vi "LogLoop_HDF5_20190307.vi"(8 "error in":errorcluster, 11 "Queue in":refnum<queue>) -> (0 "error out":errorcluster)   [LabVIEW 2018]
uses:
  Controls/Enums/LogLoopEnum.ctl
  Controls/Clusts/LogLoopClust.ctl
  Controls/Clusts/Config_Clust.ctl
  Controls/Clusts/UserConfig.ctl
  Controls/PathsCluster.ctl
  Controls/Clusts/FrontPanel_UserConfig.ctl
  Controls/Clusts/Inclinometer_User_Cfg.ctl
  Controls/Clusts/FP_UserTargetConfig.ctl
  Controls/Clusts/FreqShift.ctl
  Controls/Clusts/FPGA_Scale.ctl
  Controls/Enums/ScaleMeasure.ctl
  Controls/RadioButtons/FilterEnableRadio.ctl
  Controls/Enums/TargetNumber.ctl
  Controls/Clusts/HDF5_File_Refs.ctl
  <vilib>/addons/h5labview2/base/hid_t.ctl
  Controls/Clusts/ToneGroupRefsClust.ctl
  HDF5/HDF5_Tone_refs.ctl
  HDF5/HDF5_Noise_refs.ctl
  HDF5/TC_Tone_refs.ctl
  HDF5/HDF5_Validty_refs.ctl
  HDF5/HDF5_Disdrometer_Refs.ctl
  HDF5/HDF5_Health_Refs.ctl
  HDF5/UPS_refs.ctl
  Controls/Clusts/WeatherRefs.ctl
  HDF5/HDF5_AI_refs.ctl
  HDF5/HDF5_Filter_refs.ctl
  HDF5/HDF5_ADAM_Refs.ctl
  HDF5/HDF5_Complex_Refs.ctl
  Controls/Clusts/LogDataClust.ctl
  Controls/Clusts/ToneLogBuffered.ctl
  Controls/Clusts/SaturationMonitorBuffer.ctl
  HDF5/TC_Data_Structure.ctl
  Controls/Clusts/AI_Clust.ctl
  HDF5/HDF5_NoiseInfoClust.ctl
  HDF5/DisdrometerData.ctl
  HDF5/DisdromterSummaryData.ctl
  Disdrometer/Disdrometer_Status_Cluster.ctl
  Controls/Clusts/WeatherDataClust.ctl
  Controls/Clusts/ValidityWeatherClust.ctl
  Controls/Clusts/TE_Data_Clust.ctl
  HDF5/HDF5_ADAM_Data.ctl
  Controls/Clusts/TimeDomainData.ctl
  Controls/Clusts/AlarmSettingsClust.ctl
  Controls/Clusts/AlarmThresh_OneChan.ctl
  Controls/Clusts/ErrorStatus.ctl
  Controls/Clusts/DigOutClust.ctl
  Controls/Clusts/Saturation_Status_Clust.ctl
  Controls/Clusts/HDF5_10HzRefs.ctl
  Controls/Clusts/TargetToneData.ctl
  Controls/Clusts/ChannelToneData.ctl
  Controls/ToneInfoClust.ctl
  Controls/Clusts/SaturationMonitor.ctl
  Controls/Clusts/All_TC_Error_and_Data.ctl
  Controls/Clusts/All_TC_Error_Status.ctl
  Controls/Clusts/All_AI_Error_and_Data.ctl
  Controls/Clusts/All_AI_Error_Status.ctl
  Controls/Clusts/UPS_Status_Clust.ctl
  Controls/Enums/FP_Loop_Enum.ctl
  Controls/Enums/DigiLoopEnum.ctl
  Controls/Enums/WatchdogTimer_Enum.ctl
  <vilib>/addons/h5labview2/file/H5F.lvlib
panel:
  out "base path 2":path
  out "WatchDogElapsed":i32[](array[numeric])
  out "Elapsed":u32
  out "#LogElements":i32
  out "LogCount":i32
  out "LogState":T1
  out "date/time string":string
  out "Enum":T1
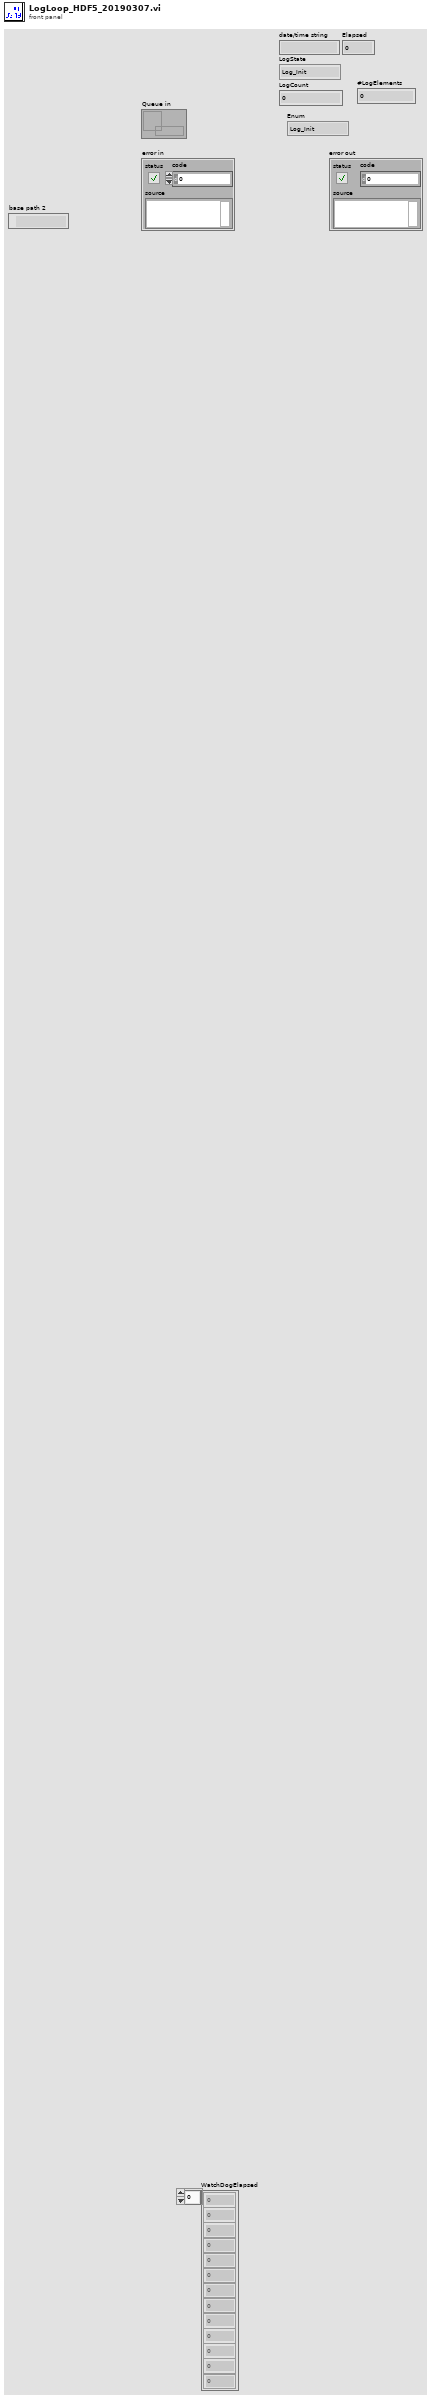
[diagram p1: front panel]
types:
  T1 = typedef "LogLoopEnum.ctl" = enum16{"Log_Init", "Log_Config", "Log_CfgAlarm", "Log_TimeDomain", "Log_Tone", "Log_NoiseTrace", "Log_NoiseSum", "Log_DO", "Log_AI", "Log_TC", "Log_Disdrom", "Log_Weather", "Log_TE", "Log_ADAM", "Log_UPS", "Log_ChkTime", "Log_Alarm", "Log_SSH", "Log_Write", "Log_Exit"}
  T2 = typedef "LogLoopClust.ctl" = cluster{"base path":path, "PathNow1":path, "PathNow2":path, "DateNow":string, "NAS path":path, "LogFiltStage":bool, "LogNoise_df_1":bool, "LogNoise_df_2":bool, "LogNoise_df_3":bool, "LogNoise_df_4":bool, "Config":T3, "HDFRefs1":T14, "HDFRefs2":T14, "LogData":T29, "AlarmCfg":T43, "DO":bool[], "AllAlarms":T45[], "Alarm Status":T46, "SaturationStatus":T47, "WeatherStatus":bool[], "10HzRefs":T48}
  T3 = typedef "Config_Clust.ctl" = cluster{"UsrCfg":T4, "FP_User":T6}
  T4 = typedef "UserConfig.ctl" = cluster{"Paths":T5, "SampleRate":dbl}
  T5 = typedef "PathsCluster.ctl" = cluster{"CfgFile":path, "LogFolder":path, "LogFile":path, "NAS path":path, "ThreshFile":path, "RedunFolder":path}
  T6 = typedef "FrontPanel_UserConfig.ctl" = cluster{"#NoiseSums":u32, "Max_df":u32, "AvgAvg":bool, "#Avg":u16, "AutoCenter":bool, "Inclin":T7, "1":T8, "2":T8, "3":T8, "4":T8, "Target to Probe":T13, "SNR_Thresh":dbl, "Paths":T5, "Connex_Location":string, "SimulateFPGA":bool, "Deadband":dbl}
  T7 = typedef "Inclinometer_User_Cfg.ctl" = cluster{"Vmin":dbl, "Vmax":dbl, "Angle_min":dbl, "Angle_max":dbl, "Offset":dbl, "Pos_Neg":bool}
  T8 = typedef "FP_UserTargetConfig.ctl" = cluster{"Cal_":T9, "Beac":T9, "Scale":T10, "Offset":fxp<+/-,16,16>, "Scale_Noise":fxp<+/-,30,30>, "Scale_Step1":fxp<+/-,17,17>, "Scale_In_RT":ext, "ScaleMeas":fxp<+/-,16,1>, "FreqsToRemove":i32[], "Width":i32[], "ScaleMeasEnum":T11, "FilterEnab":T12}
  T9 = typedef "FreqShift.ctl" = cluster{"Fine":dbl, "Coarse_":dbl}
  T10 = typedef "FPGA_Scale.ctl" = cluster{"Step4":fxp<+/-,23,23>, "Step5":fxp<+/-,23,23>, "Step6":fxp<+/-,23,23>, "Step7":fxp<+/-,23,23>}
  T11 = typedef "ScaleMeasure.ctl" = enum16{"1", "10", "50", "42"}
  T12 = typedef "FilterEnableRadio.ctl" = enum32{"None", "Step 1", "Frequency Shift", "Step 4", "Step 5", "Step 6", "Step 7"}
  T13 = typedef "TargetNumber.ctl" = enum16{"1", "2", "3", "4"}
  T14 = typedef "HDF5_File_Refs.ctl" = cluster{"File":T15, "ToneRefs":T16[], "NoiseRefs":T18[], "TC_Refs":T19, "ValidRefs":T20, "DisdromRefs":T21, "TE_Refs":T22, "UPS_Refs_Deprecated":T23, "Weath_Refs":T24, "AI_Refs":T25, "Filter_Refs":T26, "ADAM_Refs":T27, "Complex":T28[]}
  T15 = typedef "hid_t.ctl" = i32
  T16 = typedef "ToneGroupRefsClust.ctl" = cluster{"Group_ref":T15, "Cal":T17, "Beac":T17, "CalZoom_dSet":T15, "BeacZoom_dSet":T15}
  T17 = typedef "HDF5_Tone_refs.ctl" = cluster{"TimeString_dset":T15, "TImeStamp_dset":T15, "SNR_dset":T15, "MaxValue_dset":T15, "PeakLoc_dset":T15, "df_dset":T15, "Phase_dset":T15, "DeltaPhase_dset":T15, "Downshift_dset":T15}
  T18 = typedef "HDF5_Noise_refs.ctl" = cluster{"Group_ref":T15, "TimeString_dset":T15, "TimeStamp_dset":T15, "TimeStamp_df_dset":T15, "df_dset":T15, "sum_dset":T15, "SumdSpectrum_dset":T15}
  T19 = typedef "TC_Tone_refs.ctl" = cluster{"Group_ref":T15, "TimeString_dset":T15, "TimeStamp_dset":T15, "TC0_LP1_Hi":T15, "TC1_LP1_MidHi":T15, "TC2_LP1_Mid":T15, "TC3_LP1_LoMid":T15, "TC4_LP1_Lo":T15, "TC5_LP2_Hi":T15, "TC6_LP2_MidHi":T15, "TC7_LP2_Mid":T15, "TC8_LP2_LoMid":T15, "TC9_LP2_Lo":T15, "TC10_HVAC_Cond_In":T15, "TC11_HVAC_Cond_Out":T15, "TC12_Gen_Exhaust":T15, "TC13_Tamb_Inter":T15}
  T20 = typedef "HDF5_Validty_refs.ctl" = cluster{"Group_ref":T15, "Weath_Valid_dset":T15, "Disdr_Valid_dset":T15, "Saturat_dset":T15, "Alarm_Valid_dset":T15, "Time_Valid_dset":T15, "Time_AlarmChange_dset":T15, "Alarm_Source_dset":T15}
  T21 = typedef "HDF5_Disdrometer_Refs.ctl" = cluster{"BasicGroup_ref":T15, "TimeStamp_dset":T15, "TotalRainRate_dset":T15, "Liquid_dset":T15, "Solid_dset":T15, "TotalRain_dset":T15, "Visibility_dset":T15, "RadarReflect_dset":T15, "MaxDiam_dset":T15, "MeasdParticles_dset":T15, "ParticlMinSpeed_dset":T15, "ParticlMaxSpeed_dset":T15, "ParticlMinDiam_dset":T15, "NonHydrParticls_dset":T15, "NonHydrVolum_dset":T15, "UnknownParticls_dset":T15, "UnknownVolum_dset":T15, "HydromType_dset":T15, "SpectGroup_ref":T15, "Spectrum_dset":T15, "Status_dset_deprecated":T15}
  T22 = typedef "HDF5_Health_Refs.ctl" = cluster{"Group_ref":T15, "TE_Temp1_dset":T15, "TE_Outp1_dset":T15, "TE_Temp2_dset":T15, "TE_Outp2_dset":T15, "TE_Temp3_dset":T15, "TE_Outp3_dset":T15, "TimeStamp":T15}
  T23 = typedef "UPS_refs.ctl" = cluster{"Group_ref":T15, "TimeString_dset":T15, "TimeStamp_dset":T15, "V_dset":T15, "A_dset":T15, "Hz_dset":T15, "W_dset":T15, "%_dset":T15}
  T24 = typedef "WeatherRefs.ctl" = cluster{"Group_ref":T15, "TimeString_dset":T15, "TimeStamp_dset ":T15, "WindSpd_dset":T15, "WindGusts_dset":T15, "WindDir_dset":T15, "WindDirSTD_dset":T15, "Temp_dset":T15, "Humidity_dset":T15, "Pressure_dset":T15, "RainRate_dset":T15, "RainFall_dset":T15}
  T25 = typedef "HDF5_AI_refs.ctl" = cluster{"Group_ref":T15, "TimeString_dset":T15, "TimeStamp_dset":T15, "AI0_dset":T15, "AI1_dset":T15, "AI2_dset":T15, "AI3_dset":T15, "AI4_dset":T15, "AI5_dset":T15, "AI6_dset":T15, "AI16_dset":T15, "AI17_dset":T15, "AI18_dset":T15, "AzStdDev_dset":T15, "AI19_dset":T15, "ElStdDev_dset":T15, "BlowerPwr_dset":T15}
  T26 = typedef "HDF5_Filter_refs.ctl" = cluster{"Filter_Group_ref":T15, "TimeStamp_dset":T15, "Filter_dset":T15}
  T27 = typedef "HDF5_ADAM_Refs.ctl" = cluster{"Group_ref":T15, "ADAM_CoPol_dset":T15, "ADAM_XPol_dset":T15, "ADAM_Noise_dset":T15, "ADAM_CalBox_dset":T15, "TimeStamp":T15}
  T28 = typedef "HDF5_Complex_Refs.ctl" = cluster{"Group_ref":T15, "TImeStamp_dset":T15, "PwrSpect_dset":T15, "ISpect_dset":T15, "QSpect_dset":T15}
  T29 = typedef "LogDataClust.ctl" = cluster{"Tone":T30[], "TCData":T32, "AI":T33, "NoiseTrace":cluster{"Target":T13, "NoiseTrace":dbl[]}[], "NoiseInfo":cluster{"Target":T13, "HDF5_NoiseInfo":T34}[], "Disdrom":T35[], "Weath":T38[], "TE":T40, "ADAM":T41, "TimeDomain":T42[]}
  T30 = typedef "ToneLogBuffered.ctl" = cluster{"Count":i32, "CalVal":sgl[], "CalLoc":i32[], "BeacVal":sgl[], "BeacLoc":i32[], "BeacShift":i32[], "Enum":T13, "df":dbl, "PwrSpectr":sgl[][], "ISpectr":sgl[][], "QSpectr":sgl[][], "Time":timestamp[], "SNR":sgl[], "AboveThresh":bool[], "10Hz_PeakVal":dbl[], "Phase":sgl[], "DeltaPhase":dbl[], "Saturat":T31, "10MHz":bool}
  T31 = typedef "SaturationMonitorBuffer.ctl" = cluster{"Meas":bool[], "Stage1":bool[], "Stage4":bool[], "Stage5":bool[], "Stage6":bool[], "Stage7":bool[]}
  T32 = typedef "TC_Data_Structure.ctl" = cluster{"TimeStamp":dbl, "TimeString":string, "TC0_LP1_Hi":dbl, "TC1_LP1_MidHi":dbl, "TC2_LP1_Mid":dbl, "TC3_LP1_LoMid":dbl, "TC4_LP1_Lo":dbl, "TC5_LP2_Hi":dbl, "TC6_LP2_MidHi":dbl, "TC7_LP2_Mid":dbl, "TC8_LP2_LoMid":dbl, "TC9_LP2_Lo":dbl, "TC10_HVAC_Cond_In":dbl, "TC11_HVAC_Cond_Out":dbl, "TC12_Gen_Exhaust":dbl, "TC13_Amb_Inter":dbl, "TC14_Unused":dbl, "TC15_Unused":dbl, "TC16_Unused":dbl, "TC17_Unused":dbl, "TC18_Unused":dbl, "TC19_Unused":dbl, "TC20_Unused":dbl, "TC21_Unused":dbl, "TC22_Unused":dbl, "TC23_Unused":dbl, "TC24_Unused":dbl, "TC25_Unused":dbl, "TC26_Unused":dbl, "TC27_Unused":dbl, "TC28_Unused":dbl, "TC29_Unused":dbl, "TC30_Unused":dbl, "TC31_Unused":dbl}
  T33 = typedef "AI_Clust.ctl" = cluster{"TimeString":string, "Time Stamp":dbl, "AI0_Unused":dbl, "AI1_-5V":dbl, "AI2_+5V":dbl, "AI3_+6V":dbl, "AI4_+12V":dbl, "AI5_+15V":dbl, "AI6_+28V":dbl, "AI7_Unused":dbl, "Ai16_72GHz_CalPower":dbl, "Ai17_84GHz_CalPower":dbl, "Ai18_InclinAz":dbl, "Ai19_InclinEl":dbl, "Ai20_BlowerPwr":dbl, "Ai21_Unused":dbl, "Ai22_Unused":dbl, "Ai23_Unused":dbl, "InclinA_StdDev":dbl, "InclinB_StdDev":dbl, "InclinAz_Unfilt":dbl, "InclinEl_Unfilt":dbl}
  T34 = typedef "HDF5_NoiseInfoClust.ctl" = cluster{"Timestring":string, "Timestamp":dbl, "df":dbl, "Sum":dbl}
  T35 = typedef "DisdrometerData.ctl" = cluster{"Spectrum Data":i16[], "DisdromSummary":T36, "Status":T37}
  T36 = typedef "DisdromterSummaryData.ctl" = cluster{"current time":dbl, "Timestamp":dbl, "Total Rain Rate":dbl, "Liquid Rain Rate":dbl, "Solid Rain Rate":dbl, "Total Rainfall":dbl, "Visibility":dbl, "Radar Reflectivity":dbl, "Max Diameter Hail":dbl, "Measured Particles":i32, "Particle Min Speed":i16, "Particle Max Speed":i16, "Particle Min Diam":i16, "NonHydr Particles":i16, "NonHydr Volume":dbl, "Unkn Particles":i16, "Unkn Volume":dbl, "HydroType":i8}
  T37 = typedef "Disdrometer_Status_Cluster.ctl" = cluster{"Laser":bool, "Signal":bool, "LaserTemp_Analog":bool, "LaserTemp_Digital":bool, "LaserCurrent_Analog":bool, "LaserCurrent_Digital":bool, "SensorSupply":bool, "HeatLaserHead":bool, "HeatReceiverHead":bool, "TempSensor":bool, "HeatSupply":bool, "HeatHousing":bool, "HeatHeads":bool, "HeatCarriers":bool, "OutputLaserPower":bool, "Checksum":bool, "StatusInt":u16}
  T38 = typedef "WeatherDataClust.ctl" = cluster{"TimeString":string, "Timestamp":dbl, "Wind Speed":sgl, "Wind Gusts":sgl, "Wind Dir":sgl, "Wind Dir STD":sgl, "Temperature":sgl, "Humidity":sgl, "Pressure":sgl, "Rain Rate":i16, "Rain Fall":sgl, "Status":T39}
  T39 = typedef "ValidityWeatherClust.ctl" = cluster{"Temp_OutOfBounds":bool, "Temp_IncrSTD":bool, "Temp_Oth":bool, "BarPress_OutOfBounds":bool, "BarPress_IncrSTD":bool, "BarPress_Change":bool, "BarPress_Other":bool, "Humid_OutOfBounds":bool, "Humid_IncrSTD":bool, "Humid_Other":bool, "Wind__Spd_OutOfBounds":bool, "Wind_Dir_OutOfBounds":bool, "RainBuck_OutOfBounds":bool, "RainBuck_Disdrom":bool, "Disdrom_RainBuck":bool, "Placeholder":bool}
  T40 = typedef "TE_Data_Clust.ctl" = cluster{"TimeString":string, "TimeStamp":dbl, "Temp":dbl, "Output":dbl, "Temp 2":dbl, "Output 2":dbl, "Temp 3":dbl, "Output 3":dbl}
  T41 = typedef "HDF5_ADAM_Data.ctl" = cluster{"Timestamp":dbl, "Time string":string, "Fault 1":bool, "Fault 2":bool, "Fault 3":bool, "Fault 4":bool, "Fault 5":bool, "Fault 6":bool, "Value 1":dbl, "Value 2":dbl, "Value 3":dbl, "Value 4":dbl, "Value 5":dbl, "Value 6":dbl}
  T42 = typedef "TimeDomainData.ctl" = cluster{"CalTimeVal":dbl[], "CalTimeCount":u32[], "Enum":T13}
  T43 = typedef "AlarmSettingsClust.ctl" = cluster{"TC13":T44, "AI1":T44, "AI2":T44, "AI3":T44, "AI4":T44, "AI5":T44, "AI6":T44, "AI18":T44, "AI19":T44, "TE1":T44, "TE2":T44, "TE3":T44, "ADAM1":T44, "ADAM2":T44, "ADAM3":T44, "ADAM4":T44, "72CoBeacFreq":T44, "72CoCalFreq":T44, "84CoBeacFreq":T44, "84CoCalFreq":T44, "72Co_CalTonePwr":T44, "72X_CalTonePwr":T44, "84Co_CalTonePwr":T44, "84X_CalTonePwr":T44}
  T44 = typedef "AlarmThresh_OneChan.ctl" = cluster{"Enbl":bool, "ErrsAndWarns":cluster{dbl, dbl, dbl, dbl}}
  T45 = typedef "ErrorStatus.ctl" = cluster{"RX?":bool, "Warn":bool, "Error":bool, "Enabl":bool, "Source":string}
  T46 = typedef "DigOutClust.ctl" = cluster{"Green":bool, "Rx_Yell":bool, "Cx_Yell":bool, "Red":bool, "Source":string}
  T47 = typedef "Saturation_Status_Clust.ctl" = cluster{"84":bool[], "72":bool[]}
  T48 = typedef "HDF5_10HzRefs.ctl" = cluster{"72Co_dset":T15, "84Co_dset":T15, "FileRef":T15}
  T49 = typedef "All_TC_Error_and_Data.ctl" = cluster{"TCData":T32, "All_TC_ErrorStatus":T50}
  T50 = typedef "All_TC_Error_Status.ctl" = cluster{"TC 0":T45, "TC 1":T45, "TC 2":T45, "TC 3":T45, "TC 4":T45, "TC 5":T45, "TC 6":T45, "TC 7":T45, "TC 8":T45, "TC 9":T45, "TC 10":T45, "TC 11":T45, "TC 12":T45, "TC 13":T45, "TC 14":T45, "TC 15":T45, "TC 16":T45, "TC 17":T45, "TC 18":T45, "TC 19":T45, "TC 20":T45}
  T51 = typedef "All_AI_Error_and_Data.ctl" = cluster{"AI":T33, "AllErrorStatus":T52}
  T52 = typedef "All_AI_Error_Status.ctl" = cluster{"AI 0":T45, "AI 1":T45, "AI 2":T45, "AI 3":T45, "AI 4":T45, "AI 5":T45, "AI 6":T45, "AI 7":T45, "AI 16":T45, "AI 17":T45, "AI 18":T45, "AI 19":T45, "AI 20":T45, "AI 21":T45, "AI 22":T45, "AI 23":T45}
  T53 = typedef "UPS_Status_Clust.ctl" = cluster{"Prsnt?":bool, "V":dbl, "A":dbl, "Hz":dbl, "W":dbl, "%":dbl, "TimeStamp":dbl, "TimeString":string}
  T54 = typedef "WatchdogTimer_Enum.ctl" = enum16{"ResetAll", "CheckAll", "HW1", "HW2", "Tones", "FP", "Noise", "Log", "TCP", "AI", "TC", "ADAM", "Disdrom", "TE", "Weather"}
  T55 = typedef "TargetToneData.ctl" = cluster{"Cal":T56, "Beac":T56, "Time":timestamp[], "Saturat":T58}
  T56 = typedef "ChannelToneData.ctl" = cluster{"Shift_":dbl, "Peak_ToFPGA":dbl, "MaxValue":dbl, "MaxIndex":i32, "Tone":T57, "TimeDomainI":ext[], "TimeDomainQ":ext[], "PwrSpectrum":dbl[], "RunningAvgFreq":dbl, "ISpectPos":dbl[], "ISpectNeg":dbl[], "QSpectPos":dbl[], "QSpectNeg":dbl[], "10Hz_PwrSpectr":dbl[][], "SNR":dbl, "AliasWarn":bool, "10Hz_Peak":dbl[], "ISpect+-":dbl[], "QSpect+-":dbl[], "TimeStamp":timestamp, "I_Index":ext[], "Q_Index":ext[], "10MHz":bool}
  T57 = typedef "ToneInfoClust.ctl" = cluster{"PkLocTrak":dbl, "PkLocDisp":dbl, "df_":dbl, "ZoomPwr":dbl[], "Phase":dbl, "PhaseOld":dbl, "AboveThresh?":bool, "MaxI":dbl, "MaxQ":dbl, "median":dbl, "ISpect":dbl[], "QSpect":dbl[], "DeltaPhase":dbl}
  T58 = typedef "SaturationMonitor.ctl" = cluster{"MeasMean0":dbl, "MeasMean1":dbl, "MeasMax":dbl, "1_Max":dbl, "4_Max":dbl, "5_Max":dbl, "6_Max":dbl, "7_Max":dbl}
  T59 = typedef "FP_Loop_Enum.ctl" = enum16{"FP_Init", "FP_Scale", "FP_Tone", "FP_Noise", "FP_Probes", "FP_PXI", "FP_AI", "FP_TC", "FP_PWR_Hist", "FP_Alarm", "FP_Exit"}
  T60 = typedef "AlarmDisplay.ctl" = cluster{"Alarms":T46, "SerialMeas":T61, "AllAlarms":T45[], "Elapsed_SNR_Timer":dbl, "Saturation":T47}
  T61 = typedef "SerialMeasurements_Clust.ctl" = cluster{"TE_Air":dbl, "TE_Bottom":dbl, "TE_Front":dbl, "ADAM-Co":dbl, "ADAM-XPol":dbl, "ADAM-CalEncl":dbl, "ADAM-Noise":dbl}
  T62 = typedef "DigiLoopEnum.ctl" = enum16{"Dig_Init", "Digi_Write", "Digi_Exit"}
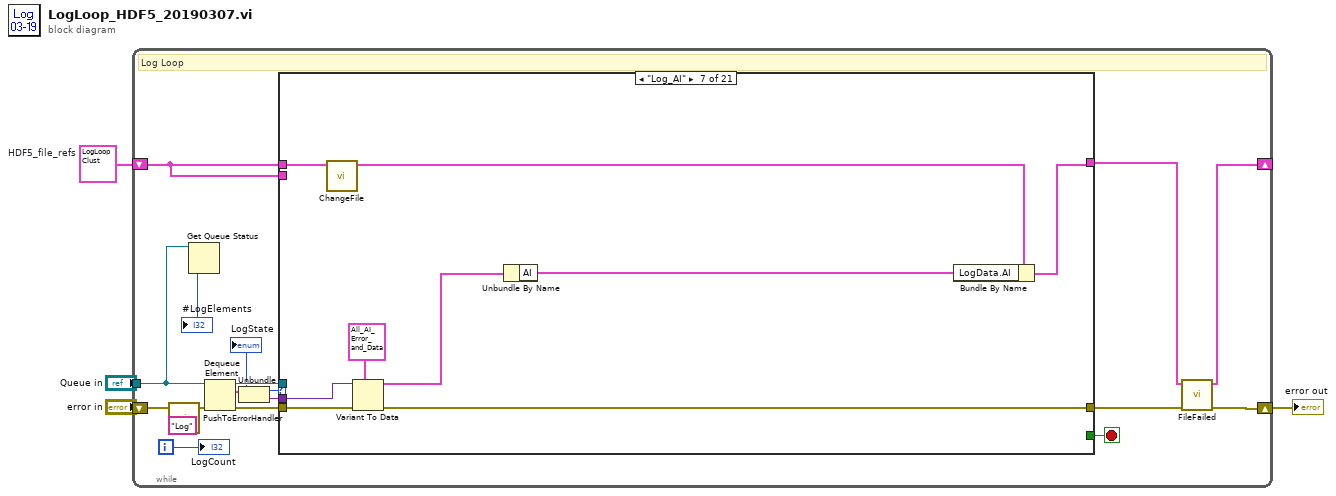
[diagram p0: block diagram]
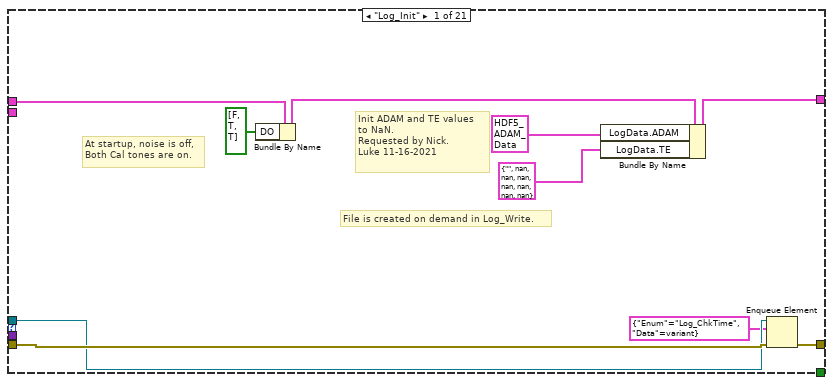
[diagram p2: hidden frame]
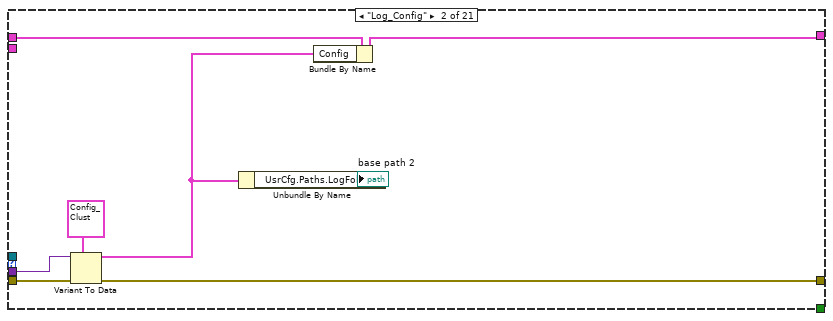
[diagram p3: hidden frame]
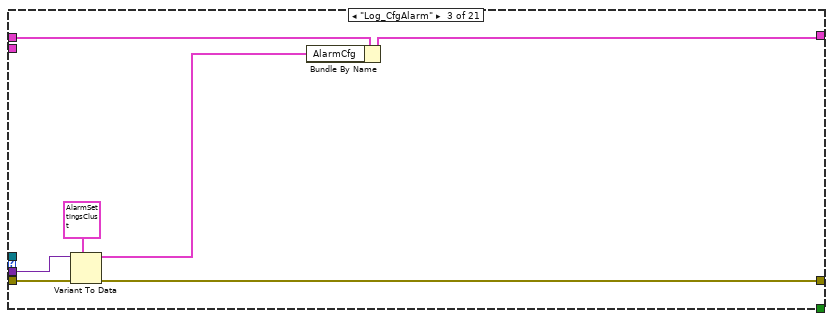
[diagram p4: hidden frame]
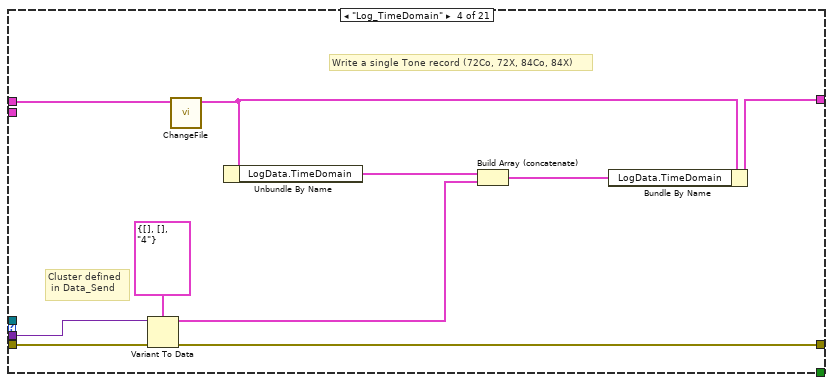
[diagram p5: hidden frame]
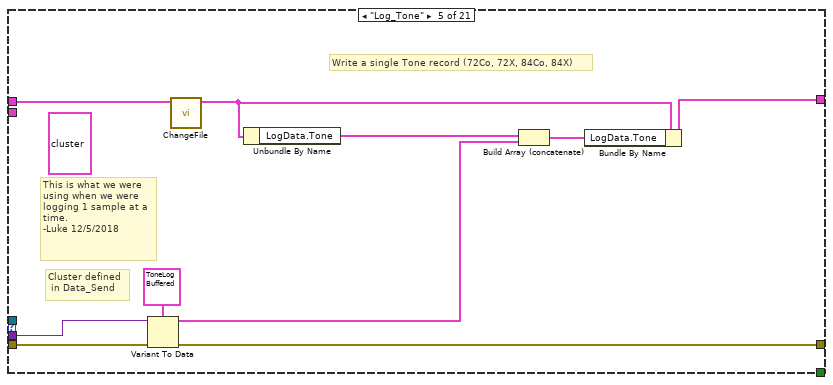
[diagram p6: hidden frame]
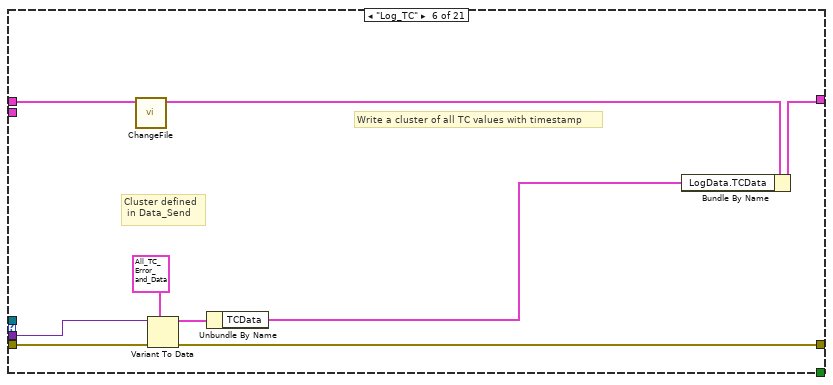
[diagram p7: hidden frame]
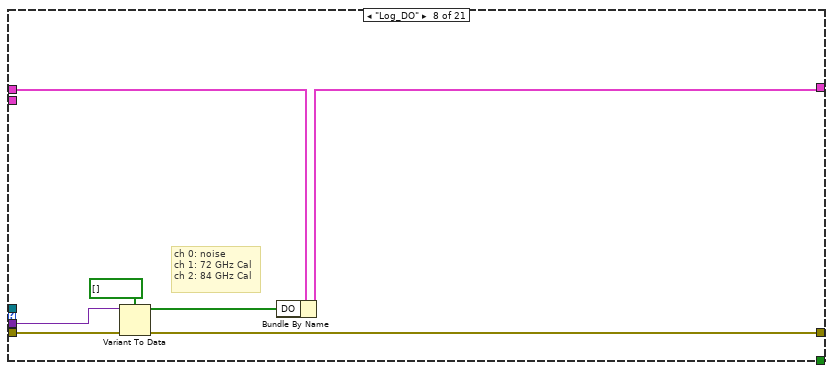
[diagram p8: hidden frame]
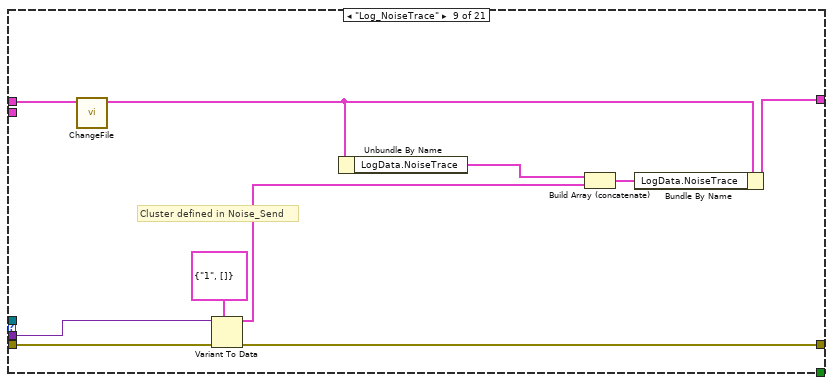
[diagram p9: hidden frame]
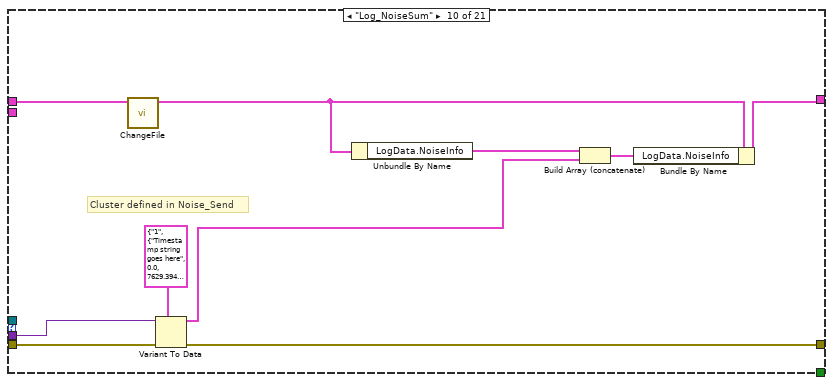
[diagram p10: hidden frame]
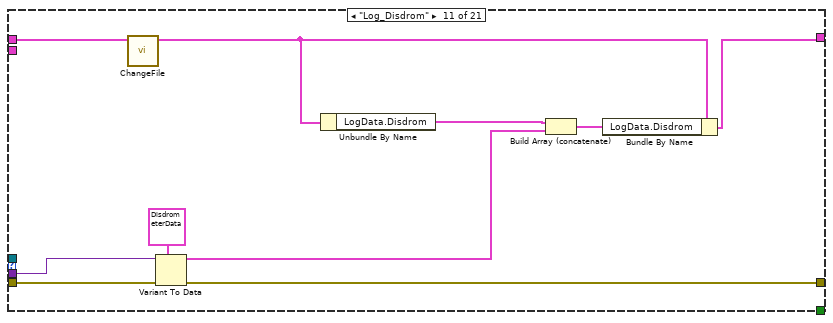
[diagram p11: hidden frame]
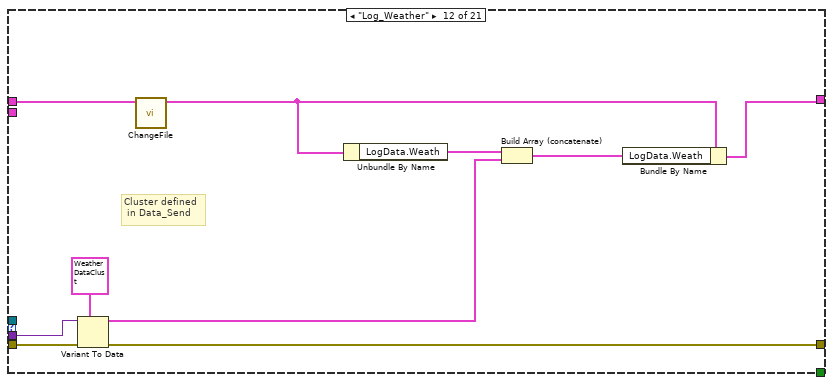
[diagram p12: hidden frame]
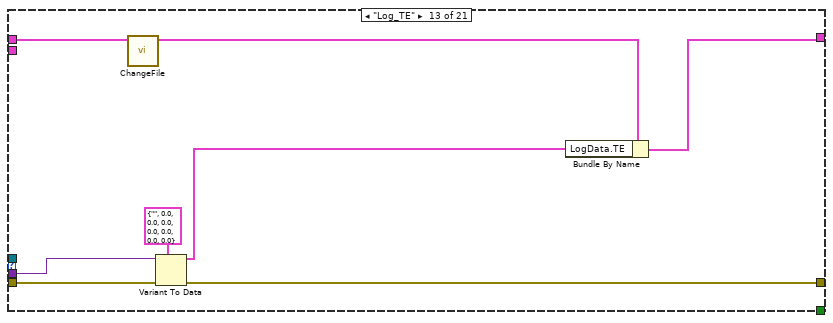
[diagram p13: hidden frame]
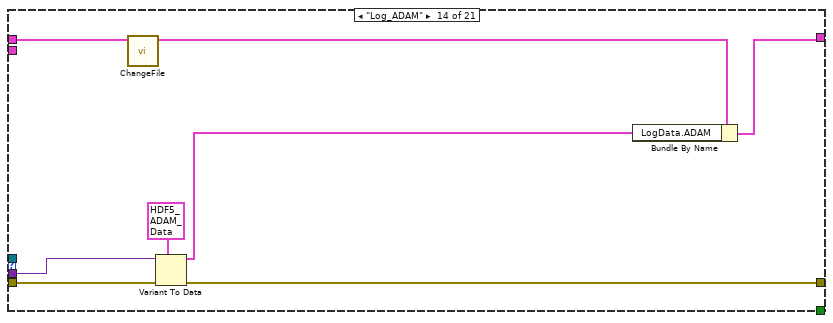
[diagram p14: hidden frame]
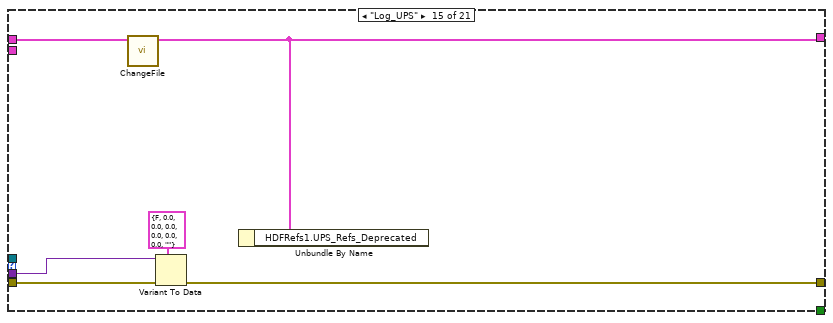
[diagram p15: hidden frame]
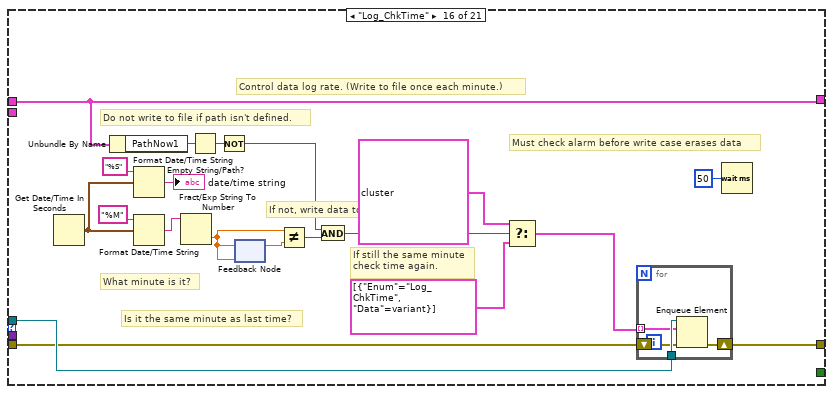
[diagram p16: hidden frame]
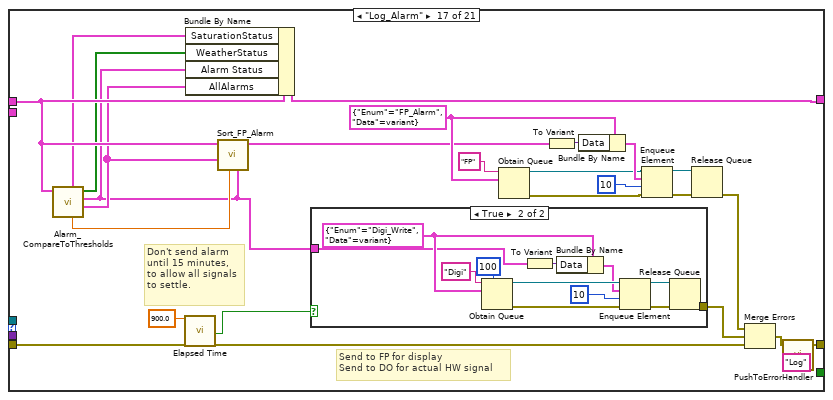
[diagram p17: hidden frame]
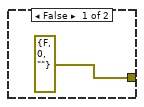
[diagram p18: hidden frame]
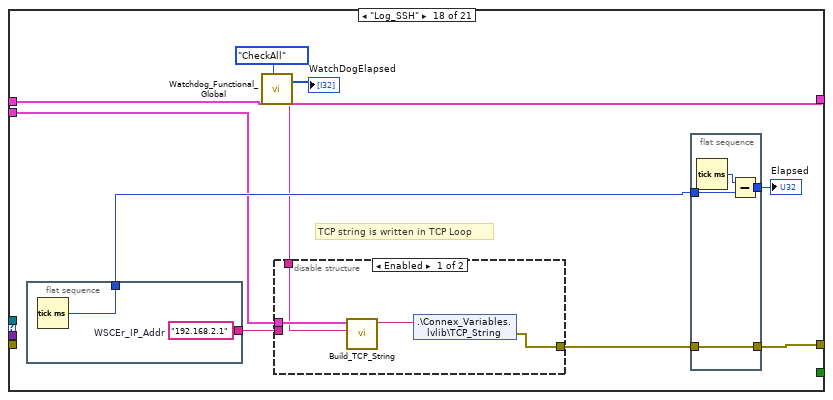
[diagram p19: hidden frame]
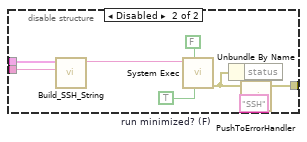
[diagram p20: hidden frame]
diagram:
  w2 = T2 {"base path"=path "", "PathNow1"=path "", "PathNow2"=path "", "DateNow"="", "NAS path"=path "", "LogFiltStage"=FALSE, "LogNoise_df_1"=FALSE, "LogNoise_df_2"=FALSE, "LogNoise_df_3"=FALSE, "LogNoise_df_4"=FALSE, "Config"={"UsrCfg"={"Paths"={"CfgFile"=path "", "LogFolder"=path "", "LogFile"=path "", "NAS path"=path "", "ThreshFile"=path "", "RedunFolder"=path ""}, "SampleRate"=0.0}, "FP_User"={"#NoiseSums"=0, "Max_df"=0, "AvgAvg"=FALSE, "#Avg"=0, "AutoCenter"=FALSE, "Inclin"={"Vmin"=0.0, "Vmax"=0.0, "Angle_min"=0.0, "Angle_max"=0.0, "Offset"=0.0, "Pos_Neg"=FALSE}, "1"={"Cal_"={"Fine"=0.0, "Coarse_"=0.0}, "Beac"={"Fine"=0.0, "Coarse_"=0.0}, "Scale"={"Step4"=0.0, "Step5"=0.0, "Step6"=0.0, "Step7"=0.0}, "Offset"=0.0, "Scale_Noise"=0.0, "Scale_Step1"=0.0, "Scale_In_RT"=0.0, "ScaleMeas"=0.0, "FreqsToRemove"=[], "Width"=[], "ScaleMeasEnum"=enum."1", "FilterEnab"=enum."None"}, "2"={"Cal_"={"Fine"=0.0, "Coarse_"=0.0}, "Beac"={"Fine"=0.0, "Coarse_"=0.0}, "Scale"={"Step4"=0.0, "Step5"=0.0, "Step6"=0.0, "Step7"=0.0}, "Offset"=0.0, "Scale_Noise"=0.0, "Scale_Step1"=0.0, "Scale_In_RT"=0.0, "ScaleMeas"=0.0, "FreqsToRemove"=[], "Width"=[], "ScaleMeasEnum"=enum."1", "FilterEnab"=enum."None"}, "3"={"Cal_"={"Fine"=0.0, "Coarse_"=0.0}, "Beac"={"Fine"=0.0, "Coarse_"=0.0}, "Scale"={"Step4"=0.0, "Step5"=0.0, "Step6"=0.0, "Step7"=0.0}, "Offset"=0.0, "Scale_Noise"=0.0, "Scale_Step1"=0.0, "Scale_In_RT"=0.0, "ScaleMeas"=0.0, "FreqsToRemove"=[], "Width"=[], "ScaleMeasEnum"=enum."1", "FilterEnab"=enum."None"}, "4"={"Cal_"={"Fine"=0.0, "Coarse_"=0.0}, "Beac"={"Fine"=0.0, "Coarse_"=0.0}, "Scale"={"Step4"=0.0, "Step5"=0.0, "Step6"=0.0, "Step7"=0.0}, "Offset"=0.0, "Scale_Noise"=0.0, "Scale_Step1"=0.0, "Scale_In_RT"=0.0, "ScaleMeas"=0.0, "FreqsToRemove"=[], "Width"=[], "ScaleMeasEnum"=enum."1", "FilterEnab"=enum."None"}, "Target to Probe"=enum."1", "SNR_Thresh"=0.0, "Paths"={"CfgFile"=path "", "LogFolder"=path "", "LogFile"=path "", "NAS path"=path "", "ThreshFile"=path "", "RedunFolder"=path ""}, "Connex_Location"="", "SimulateFPGA"=FALSE, "Deadband"=0.0}}, "HDFRefs1"={"File"=0, "ToneRefs"=[], "NoiseRefs"=[], "TC_Refs"={"Group_ref"=0, "TimeString_dset"=0, "TimeStamp_dset"=0, "TC0_LP1_Hi"=0, "TC1_LP1_MidHi"=0, "TC2_LP1_Mid"=0, "TC3_LP1_LoMid"=0, "TC4_LP1_Lo"=0, "TC5_LP2_Hi"=0, "TC6_LP2_MidHi"=0, "TC7_LP2_Mid"=0, "TC8_LP2_LoMid"=0, "TC9_LP2_Lo"=0, "TC10_HVAC_Cond_In"=0, "TC11_HVAC_Cond_Out"=0, "TC12_Gen_Exhaust"=0, "TC13_Tamb_Inter"=0}, "ValidRefs"={"Group_ref"=0, "Weath_Valid_dset"=0, "Disdr_Valid_dset"=0, "Saturat_dset"=0, "Alarm_Valid_dset"=0, "Time_Valid_dset"=0, "Time_AlarmChange_dset"=0, "Alarm_Source_dset"=0}, "DisdromRefs"={"BasicGroup_ref"=0, "TimeStamp_dset"=0, "TotalRainRate_dset"=0, "Liquid_dset"=0, "Solid_dset"=0, "TotalRain_dset"=0, "Visibility_dset"=0, "RadarReflect_dset"=0, "MaxDiam_dset"=0, "MeasdParticles_dset"=0, "ParticlMinSpeed_dset"=0, "ParticlMaxSpeed_dset"=0, "ParticlMinDiam_dset"=0, "NonHydrParticls_dset"=0, "NonHydrVolum_dset"=0, "UnknownParticls_dset"=0, "UnknownVolum_dset"=0, "HydromType_dset"=0, "SpectGroup_ref"=0, "Spectrum_dset"=0, "Status_dset_deprecated"=0}, "TE_Refs"={"Group_ref"=0, "TE_Temp1_dset"=0, "TE_Outp1_dset"=0, "TE_Temp2_dset"=0, "TE_Outp2_dset"=0, "TE_Temp3_dset"=0, "TE_Outp3_dset"=0, "TimeStamp"=0}, "UPS_Refs_Deprecated"={"Group_ref"=0, "TimeString_dset"=0, "TimeStamp_dset"=0, "V_dset"=0, "A_dset"=0, "Hz_dset"=0, "W_dset"=0, "%_dset"=0}, "Weath_Refs"={"Group_ref"=0, "TimeString_dset"=0, "TimeStamp_dset "=0, "WindSpd_dset"=0, "WindGusts_dset"=0, "WindDir_dset"=0, "WindDirSTD_dset"=0, "Temp_dset"=0, "Humidity_dset"=0, "Pressure_dset"=0, "RainRate_dset"=0, "RainFall_dset"=0}, "AI_Refs"={"Group_ref"=0, "TimeString_dset"=0, "TimeStamp_dset"=0, "AI0_dset"=0, "AI1_dset"=0, "AI2_dset"=0, "AI3_dset"=0, "AI4_dset"=0, "AI5_dset"=0, "AI6_dset"=0, "AI16_dset"=0, "AI17_dset"=0, "AI18_dset"=0, "AzStdDev_dset"=0, "AI19_dset"=0, "ElStdDev_dset"=0, "BlowerPwr_dset"=0}, "Filter_Refs"={"Filter_Group_ref"=0, "TimeStamp_dset"=0, "Filter_dset"=0}, "ADAM_Refs"={"Group_ref"=0, "ADAM_CoPol_dset"=0, "ADAM_XPol_dset"=0, "ADAM_Noise_dset"=0, "ADAM_CalBox_dset"=0, "TimeStamp"=0}, "Complex"=[]}, "HDFRefs2"={"File"=0, "ToneRefs"=[], "NoiseRefs"=[], "TC_Refs"={"Group_ref"=0, "TimeString_dset"=0, "TimeStamp_dset"=0, "TC0_LP1_Hi"=0, "TC1_LP1_MidHi"=0, "TC2_LP1_Mid"=0, "TC3_LP1_LoMid"=0, "TC4_LP1_Lo"=0, "TC5_LP2_Hi"=0, "TC6_LP2_MidHi"=0, "TC7_LP2_Mid"=0, "TC8_LP2_LoMid"=0, "TC9_LP2_Lo"=0, "TC10_HVAC_Cond_In"=0, "TC11_HVAC_Cond_Out"=0, "TC12_Gen_Exhaust"=0, "TC13_Tamb_Inter"=0}, "ValidRefs"={"Group_ref"=0, "Weath_Valid_dset"=0, "Disdr_Valid_dset"=0, "Saturat_dset"=0, "Alarm_Valid_dset"=0, "Time_Valid_dset"=0, "Time_AlarmChange_dset"=0, "Alarm_Source_dset"=0}, "DisdromRefs"={"BasicGroup_ref"=0, "TimeStamp_dset"=0, "TotalRainRate_dset"=0, "Liquid_dset"=0, "Solid_dset"=0, "TotalRain_dset"=0, "Visibility_dset"=0, "RadarReflect_dset"=0, "MaxDiam_dset"=0, "MeasdParticles_dset"=0, "ParticlMinSpeed_dset"=0, "ParticlMaxSpeed_dset"=0, "ParticlMinDiam_dset"=0, "NonHydrParticls_dset"=0, "NonHydrVolum_dset"=0, "UnknownParticls_dset"=0, "UnknownVolum_dset"=0, "HydromType_dset"=0, "SpectGroup_ref"=0, "Spectrum_dset"=0, "Status_dset_deprecated"=0}, "TE_Refs"={"Group_ref"=0, "TE_Temp1_dset"=0, "TE_Outp1_dset"=0, "TE_Temp2_dset"=0, "TE_Outp2_dset"=0, "TE_Temp3_dset"=0, "TE_Outp3_dset"=0, "TimeStamp"=0}, "UPS_Refs_Deprecated"={"Group_ref"=0, "TimeString_dset"=0, "TimeStamp_dset"=0, "V_dset"=0, "A_dset"=0, "Hz_dset"=0, "W_dset"=0, "%_dset"=0}, "Weath_Refs"={"Group_ref"=0, "TimeString_dset"=0, "TimeStamp_dset "=0, "WindSpd_dset"=0, "WindGusts_dset"=0, "WindDir_dset"=0, "WindDirSTD_dset"=0, "Temp_dset"=0, "Humidity_dset"=0, "Pressure_dset"=0, "RainRate_dset"=0, "RainFall_dset"=0}, "AI_Refs"={"Group_ref"=0, "TimeString_dset"=0, "TimeStamp_dset"=0, "AI0_dset"=0, "AI1_dset"=0, "AI2_dset"=0, "AI3_dset"=0, "AI4_dset"=0, "AI5_dset"=0, "AI6_dset"=0, "AI16_dset"=0, "AI17_dset"=0, "AI18_dset"=0, "AzStdDev_dset"=0, "AI19_dset"=0, "ElStdDev_dset"=0, "BlowerPwr_dset"=0}, "Filter_Refs"={"Filter_Group_ref"=0, "TimeStamp_dset"=0, "Filter_dset"=0}, "ADAM_Refs"={"Group_ref"=0, "ADAM_CoPol_dset"=0, "ADAM_XPol_dset"=0, "ADAM_Noise_dset"=0, "ADAM_CalBox_dset"=0, "TimeStamp"=0}, "Complex"=[]}, "LogData"={"Tone"=[], "TCData"={"TimeStamp"=0.0, "TimeString"="", "TC0_LP1_Hi"=0.0, "TC1_LP1_MidHi"=0.0, "TC2_LP1_Mid"=0.0, "TC3_LP1_LoMid"=0.0, "TC4_LP1_Lo"=0.0, "TC5_LP2_Hi"=0.0, "TC6_LP2_MidHi"=0.0, "TC7_LP2_Mid"=0.0, "TC8_LP2_LoMid"=0.0, "TC9_LP2_Lo"=0.0, "TC10_HVAC_Cond_In"=0.0, "TC11_HVAC_Cond_Out"=0.0, "TC12_Gen_Exhaust"=0.0, "TC13_Amb_Inter"=0.0, "TC14_Unused"=0.0, "TC15_Unused"=0.0, "TC16_Unused"=0.0, "TC17_Unused"=0.0, "TC18_Unused"=0.0, "TC19_Unused"=0.0, "TC20_Unused"=0.0, "TC21_Unused"=0.0, "TC22_Unused"=0.0, "TC23_Unused"=0.0, "TC24_Unused"=0.0, "TC25_Unused"=0.0, "TC26_Unused"=0.0, "TC27_Unused"=0.0, "TC28_Unused"=0.0, "TC29_Unused"=0.0, "TC30_Unused"=0.0, "TC31_Unused"=0.0}, "AI"={"TimeString"="", "Time Stamp"=0.0, "AI0_Unused"=0.0, "AI1_-5V"=0.0, "AI2_+5V"=0.0, "AI3_+6V"=0.0, "AI4_+12V"=0.0, "AI5_+15V"=0.0, "AI6_+28V"=0.0, "AI7_Unused"=0.0, "Ai16_72GHz_CalPower"=0.0, "Ai17_84GHz_CalPower"=0.0, "Ai18_InclinAz"=0.0, "Ai19_InclinEl"=0.0, "Ai20_BlowerPwr"=0.0, "Ai21_Unused"=0.0, "Ai22_Unused"=0.0, "Ai23_Unused"=0.0, "InclinA_StdDev"=0.0, "InclinB_StdDev"=0.0, "InclinAz_Unfilt"=0.0, "InclinEl_Unfilt"=0.0}, "NoiseTrace"=[], "NoiseInfo"=[], "Disdrom"=[], "Weath"=[], "TE"={"TimeString"="", "TimeStamp"=0.0, "Temp"=0.0, "Output"=0.0, "Temp 2"=0.0, "Output 2"=0.0, "Temp 3"=0.0, "Output 3"=0.0}, "ADAM"={"Timestamp"=0.0, "Time string"="", "Fault 1"=FALSE, "Fault 2"=FALSE, "Fault 3"=FALSE, "Fault 4"=FALSE, "Fault 5"=FALSE, "Fault 6"=FALSE, "Value 1"=0.0, "Value 2"=0.0, "Value 3"=0.0, "Value 4"=0.0, "Value 5"=0.0, "Value 6"=0.0}, "TimeDomain"=[]}, "AlarmCfg"={"TC13"={"Enbl"=FALSE, "ErrsAndWarns"={0.0, 0.0, 0.0, 0.0}}, "AI1"={"Enbl"=FALSE, "ErrsAndWarns"={0.0, 0.0, 0.0, 0.0}}, "AI2"={"Enbl"=FALSE, "ErrsAndWarns"={0.0, 0.0, 0.0, 0.0}}, "AI3"={"Enbl"=FALSE, "ErrsAndWarns"={0.0, 0.0, 0.0, 0.0}}, "AI4"={"Enbl"=FALSE, "ErrsAndWarns"={0.0, 0.0, 0.0, 0.0}}, "AI5"={"Enbl"=FALSE, "ErrsAndWarns"={0.0, 0.0, 0.0, 0.0}}, "AI6"={"Enbl"=FALSE, "ErrsAndWarns"={0.0, 0.0, 0.0, 0.0}}, "AI18"={"Enbl"=FALSE, "ErrsAndWarns"={0.0, 0.0, 0.0, 0.0}}, "AI19"={"Enbl"=FALSE, "ErrsAndWarns"={0.0, 0.0, 0.0, 0.0}}, "TE1"={"Enbl"=FALSE, "ErrsAndWarns"={0.0, 0.0, 0.0, 0.0}}, "TE2"={"Enbl"=FALSE, "ErrsAndWarns"={0.0, 0.0, 0.0, 0.0}}, "TE3"={"Enbl"=FALSE, "ErrsAndWarns"={0.0, 0.0, 0.0, 0.0}}, "ADAM1"={"Enbl"=FALSE, "ErrsAndWarns"={0.0, 0.0, 0.0, 0.0}}, "ADAM2"={"Enbl"=FALSE, "ErrsAndWarns"={0.0, 0.0, 0.0, 0.0}}, "ADAM3"={"Enbl"=FALSE, "ErrsAndWarns"={0.0, 0.0, 0.0, 0.0}}, "ADAM4"={"Enbl"=FALSE, "ErrsAndWarns"={0.0, 0.0, 0.0, 0.0}}, "72CoBeacFreq"={"Enbl"=FALSE, "ErrsAndWarns"={0.0, 0.0, 0.0, 0.0}}, "72CoCalFreq"={"Enbl"=FALSE, "ErrsAndWarns"={0.0, 0.0, 0.0, 0.0}}, "84CoBeacFreq"={"Enbl"=FALSE, "ErrsAndWarns"={0.0, 0.0, 0.0, 0.0}}, "84CoCalFreq"={"Enbl"=FALSE, "ErrsAndWarns"={0.0, 0.0, 0.0, 0.0}}, "72Co_CalTonePwr"={"Enbl"=FALSE, "ErrsAndWarns"={0.0, 0.0, 0.0, 0.0}}, "72X_CalTonePwr"={"Enbl"=FALSE, "ErrsAndWarns"={0.0, 0.0, 0.0, 0.0}}, "84Co_CalTonePwr"={"Enbl"=FALSE, "ErrsAndWarns"={0.0, 0.0, 0.0, 0.0}}, "84X_CalTonePwr"={"Enbl"=FALSE, "ErrsAndWarns"={0.0, 0.0, 0.0, 0.0}}}, "DO"=[], "AllAlarms"=[], "Alarm Status"={"Green"=FALSE, "Rx_Yell"=FALSE, "Cx_Yell"=FALSE, "Red"=FALSE, "Source"=""}, "SaturationStatus"={"84"=[], "72"=[]}, "WeatherStatus"=[], "10HzRefs"={"72Co_dset"=0, "84Co_dset"=0, "FileRef"=0}}  # HDF5_file_refs
  n1 = while {
    tunnel: "Queue in" -> [w8]
    shift-right: [w14] -> w3
    shift-left: "error in" -> [w18]
    shift-right: [w13] -> _
    shift-left: w2 -> [w5]
    i -> [w9]
    stop <- w15 stop-if-true
    # "Log Loop"
    n2 = call "PushToErrorHandler.vi"("ErrorIn"=w18, "ErrorLocation"="Log") -> ("ErrorOut"=w20:errorcluster)  [unwired: 5 in]
    n3 = Get Queue Status(queue=w8) -> (# elements in queue=→"#LogElements":i32)  [unwired: 2 in, 7 out]
    n4 = Dequeue Element(queue=w8, error in (no error)=w20) -> (queue out=w17:refnum<queue>, element=w19:cluster{"Enum":T1, "Data":variant}, error out=w16:errorcluster)  [unwired: 1 in, 1 out]
    n5 = Unbundle(w19) -> ("Enum"=w12:T1, "Data"=w11:variant)
    "LogState" <- w12
    n6 = case shown="\"Log_AI\"" w12 {
      selector: w12 -> [_ _ _ _ _ _ _ _ _ _ _ _ _ _ _ _ _ _ _ _ w267]
      tunnel: w17 -> [w28 _ _ _ _ _ _ _ _ _ _ _ _ _ _ w172 _ _ _ w265 _]
      tunnel: w16 -> [w31 w38 w45 w56 w66 w75 w84 w90 w101 w111 w121 w131 w139 w147 w153 w171 w190 _ w251 w264 w268]
      tunnel: w11 -> [_ w36 w43 w55 w65 w74 w83 w88 w100 w110 w120 w130 w138 w146 w152 _ _ _ _ _ _]
      tunnel: [w29 w37 w44 w48 w57 w69 w78 w91 w99 w107 w117 w127 w136 w144 w148 w173 w194 w225 w248 w253 w268] -> w10
      tunnel: [_ _ _ _ _ _ _ _ _ _ _ _ _ _ _ _ _ _ _ TRUE _] -> w15
      tunnel: w5 -> [w30 w39 w46 w54 w64 w73 w82 w86 w98 w109 w119 w129 w137 w145 w151 w162 w184 w226 w247 w261 w266]
      tunnel: [w24 w34 w42 w51 w61 w71 w80 w87 w96 w106 w113 w126 w133 w141 w150 w162 w185 w226 w245 w261 w266] -> w6
      tunnel: w5 -> [_ _ _ _ _ _ _ _ _ _ _ _ _ _ _ _ _ w221 _ _ _]
      frame "Log_Init" {
        # "Init ADAM and TE values\nto NaN.\nRequested by Nick.\nLuke 11-16-2021"
        # "File is created on demand in Log_Write."
        # "At startup, noise is off,\nBoth Cal tones are on."
        n7 = Bundle By Name(cluster=w30, "DO"=bool[] [FALSE, TRUE, TRUE]) -> (w25:T2)
        n8 = Bundle By Name(cluster=w25, "LogData.ADAM"=T41 {"Timestamp"=0.0, "Time string"="", "Fault 1"=FALSE, "Fault 2"=FALSE, "Fault 3"=FALSE, "Fault 4"=FALSE, "Fault 5"=FALSE, "Fault 6"=FALSE, "Value 1"=nan, "Value 2"=nan, "Value 3"=nan, "Value 4"=nan, "Value 5"=nan, "Value 6"=nan}, "LogData.TE"=T40 {"TimeString"="", "TimeStamp"=nan, "Temp"=nan, "Output"=nan, "Temp 2"=nan, "Output 2"=nan, "Temp 3"=nan, "Output 3"=nan}) -> (w24:T2)
        n9 = Enqueue Element(queue=w28, element=cluster{"Enum":T1, "Data":variant} {"Enum"=enum."Log_ChkTime", "Data"=variant}, error in (no error)=w31) -> (error out=w29:errorcluster)  [unwired: 1 in, 2 out]
      }
      frame "Log_Config" {
        n10 = Variant To Data(error in=w38, type=T3 {"UsrCfg"={"Paths"={"CfgFile"=path "", "LogFolder"=path "", "LogFile"=path "", "NAS path"=path "", "ThreshFile"=path "", "RedunFolder"=path ""}, "SampleRate"=12500.0}, "FP_User"={"#NoiseSums"=1, "Max_df"=1, "AvgAvg"=FALSE, "#Avg"=1, "AutoCenter"=FALSE, "Inclin"={"Vmin"=0.0, "Vmax"=0.0, "Angle_min"=0.0, "Angle_max"=0.0, "Offset"=0.0, "Pos_Neg"=FALSE}, "1"={"Cal_"={"Fine"=0.000213623046875, "Coarse_"=4194303.0}, "Beac"={"Fine"=4194303.0, "Coarse_"=1.0}, "Scale"={"Step4"=10000.0, "Step5"=4194303.0, "Step6"=1.0, "Step7"=10000.0}, "Offset"=0.0, "Scale_Noise"=4194303.0, "Scale_Step1"=65535.0, "Scale_In_RT"=1.0, "ScaleMeas"=0.999969482421875, "FreqsToRemove"=[0, 1633], "Width"=[0, 1633], "ScaleMeasEnum"=enum."50", "FilterEnab"=enum."Step 1"}, "2"={"Cal_"={"Fine"=0.000213623046875, "Coarse_"=4194303.0}, "Beac"={"Fine"=0.000213623046875, "Coarse_"=4194303.0}, "Scale"={"Step4"=0.0, "Step5"=4194303.0, "Step6"=1.0, "Step7"=10000.0}, "Offset"=0.0, "Scale_Noise"=4194303.0, "Scale_Step1"=65535.0, "Scale_In_RT"=1.0, "ScaleMeas"=0.999969482421875, "FreqsToRemove"=[0, 1633], "Width"=[0, 1633], "ScaleMeasEnum"=enum."50", "FilterEnab"=enum."Step 1"}, "3"={"Cal_"={"Fine"=0.000213623046875, "Coarse_"=4194303.0}, "Beac"={"Fine"=0.000213623046875, "Coarse_"=4194303.0}, "Scale"={"Step4"=0.0, "Step5"=4194303.0, "Step6"=1.0, "Step7"=10000.0}, "Offset"=0.0, "Scale_Noise"=4194303.0, "Scale_Step1"=65535.0, "Scale_In_RT"=1.0, "ScaleMeas"=0.999969482421875, "FreqsToRemove"=[0, 1633], "Width"=[0, 1633], "ScaleMeasEnum"=enum."50", "FilterEnab"=enum."Step 1"}, "4"={"Cal_"={"Fine"=0.000213623046875, "Coarse_"=4194303.0}, "Beac"={"Fine"=0.000213623046875, "Coarse_"=4194303.0}, "Scale"={"Step4"=0.0, "Step5"=4194303.0, "Step6"=1.0, "Step7"=10000.0}, "Offset"=0.0, "Scale_Noise"=4194303.0, "Scale_Step1"=1.0, "Scale_In_RT"=10000.0, "ScaleMeas"=0.999969482421875, "FreqsToRemove"=[0, 1633], "Width"=[0, 1633], "ScaleMeasEnum"=enum."50", "FilterEnab"=enum."Step 1"}, "Target to Probe"=enum."4", "SNR_Thresh"=1.0, "Paths"={"CfgFile"=path "", "LogFolder"=path "", "LogFile"=path "", "NAS path"=path "", "ThreshFile"=path "", "RedunFolder"=path ""}, "Connex_Location"="", "SimulateFPGA"=FALSE, "Deadband"=0.0}} ("Config"), Variant=w36) -> (data=w32:T3, error out=w37:errorcluster)
        n11 = Unbundle By Name(w32) -> ("UsrCfg.Paths.LogFolder"=→"base path 2":path)
        n12 = Bundle By Name(cluster=w39, "Config"=w32) -> (w34:T2)
      }
      frame "Log_CfgAlarm" {
        n13 = Variant To Data(error in=w45, type=T43 {"TC13"={"Enbl"=FALSE, "ErrsAndWarns"={0.0, 0.0, 0.0, 0.0}}, "AI1"={"Enbl"=FALSE, "ErrsAndWarns"={0.0, 0.0, 0.0, 0.0}}, "AI2"={"Enbl"=FALSE, "ErrsAndWarns"={0.0, 0.0, 0.0, 0.0}}, "AI3"={"Enbl"=FALSE, "ErrsAndWarns"={0.0, 0.0, 0.0, 0.0}}, "AI4"={"Enbl"=FALSE, "ErrsAndWarns"={0.0, 0.0, 0.0, 0.0}}, "AI5"={"Enbl"=FALSE, "ErrsAndWarns"={0.0, 0.0, 0.0, 0.0}}, "AI6"={"Enbl"=FALSE, "ErrsAndWarns"={0.0, 0.0, 0.0, 0.0}}, "AI18"={"Enbl"=FALSE, "ErrsAndWarns"={0.0, 0.0, 0.0, 0.0}}, "AI19"={"Enbl"=FALSE, "ErrsAndWarns"={0.0, 0.0, 0.0, 0.0}}, "TE1"={"Enbl"=FALSE, "ErrsAndWarns"={0.0, 0.0, 0.0, 0.0}}, "TE2"={"Enbl"=FALSE, "ErrsAndWarns"={0.0, 0.0, 0.0, 0.0}}, "TE3"={"Enbl"=FALSE, "ErrsAndWarns"={0.0, 0.0, 0.0, 0.0}}, "ADAM1"={"Enbl"=FALSE, "ErrsAndWarns"={0.0, 0.0, 0.0, 0.0}}, "ADAM2"={"Enbl"=FALSE, "ErrsAndWarns"={0.0, 0.0, 0.0, 0.0}}, "ADAM3"={"Enbl"=FALSE, "ErrsAndWarns"={0.0, 0.0, 0.0, 0.0}}, "ADAM4"={"Enbl"=FALSE, "ErrsAndWarns"={0.0, 0.0, 0.0, 0.0}}, "72CoBeacFreq"={"Enbl"=FALSE, "ErrsAndWarns"={0.0, 0.0, 0.0, 0.0}}, "72CoCalFreq"={"Enbl"=FALSE, "ErrsAndWarns"={0.0, 0.0, 0.0, 0.0}}, "84CoBeacFreq"={"Enbl"=FALSE, "ErrsAndWarns"={0.0, 0.0, 0.0, 0.0}}, "84CoCalFreq"={"Enbl"=FALSE, "ErrsAndWarns"={0.0, 0.0, 0.0, 0.0}}, "72Co_CalTonePwr"={"Enbl"=FALSE, "ErrsAndWarns"={0.0, 0.0, 0.0, 0.0}}, "72X_CalTonePwr"={"Enbl"=FALSE, "ErrsAndWarns"={0.0, 0.0, 0.0, 0.0}}, "84Co_CalTonePwr"={"Enbl"=FALSE, "ErrsAndWarns"={0.0, 0.0, 0.0, 0.0}}, "84X_CalTonePwr"={"Enbl"=FALSE, "ErrsAndWarns"={0.0, 0.0, 0.0, 0.0}}} ("AlarmSettings"), Variant=w43) -> (data=w41:T43, error out=w44:errorcluster)
        n14 = Bundle By Name(cluster=w46, "AlarmCfg"=w41) -> (w42:T2)
      }
      frame "Log_TimeDomain" {
        # "Cluster defined\n in Data_Send"
        # "Write a single Tone record (72Co, 72X, 84Co, 84X)"
        n15 = Variant To Data(error in=w56, type=T42 {"CalTimeVal"=[], "CalTimeCount"=[], "Enum"=enum."4"} ("72co"), Variant=w55) -> (data=w47:T42, error out=w48:errorcluster)
        n16 = call "ChangeFile.vi"("LogLoopClust"=w54) -> ("LogLoopClust out"=w52:T2)  [unwired: 10 in]
        n17 = Unbundle By Name(w52) -> ("LogData.TimeDomain"=w50:T42[])
        n18 = Build Array (concatenate)(w50, w47) -> (w49:T42[])
        n19 = Bundle By Name(cluster=w52, "LogData.TimeDomain"=w49) -> (w51:T2)
      }
      frame "Log_Tone" {
        (unwired) cluster{"Target":T13, "1":T55} {"Target"=enum."1", "1"={"Cal"={"Shift_"=0.0, "Peak_ToFPGA"=-24999462.633451957, "MaxValue"=0.0, "MaxIndex"=0, "Tone"={"PkLocTrak"=0.0, "PkLocDisp"=0.0, "df_"=0.0, "ZoomPwr"=[], "Phase"=0.0, "PhaseOld"=0.0, "AboveThresh?"=FALSE, "MaxI"=0.0, "MaxQ"=0.0, "median"=0.0, "ISpect"=[], "QSpect"=[], "DeltaPhase"=0.0}, "TimeDomainI"=[], "TimeDomainQ"=array[12500 elements], "PwrSpectrum"=[], "RunningAvgFreq"=0.0, "ISpectPos"=[], "ISpectNeg"=[], "QSpectPos"=[], "QSpectNeg"=[], "10Hz_PwrSpectr"=[], "SNR"=0.0, "AliasWarn"=FALSE, "10Hz_Peak"=[], "ISpect+-"=[], "QSpect+-"=[], "TimeStamp"=timestamp(0 s since 1904-01-01), "I_Index"=array[12500 elements], "Q_Index"=array[12500 elements], "10MHz"=FALSE}, "Beac"={"Shift_"=0.0, "Peak_ToFPGA"=-24999462.633451957, "MaxValue"=0.0, "MaxIndex"=0, "Tone"={"PkLocTrak"=0.0, "PkLocDisp"=0.0, "df_"=0.0, "ZoomPwr"=[], "Phase"=0.0, "PhaseOld"=0.0, "AboveThresh?"=FALSE, "MaxI"=0.0, "MaxQ"=0.0, "median"=0.0, "ISpect"=[], "QSpect"=[], "DeltaPhase"=0.0}, "TimeDomainI"=[], "TimeDomainQ"=array[12500 elements], "PwrSpectrum"=[], "RunningAvgFreq"=0.0, "ISpectPos"=[], "ISpectNeg"=[], "QSpectPos"=[], "QSpectNeg"=[], "10Hz_PwrSpectr"=[], "SNR"=0.0, "AliasWarn"=FALSE, "10Hz_Peak"=[], "ISpect+-"=[], "QSpect+-"=[], "TimeStamp"=timestamp(0 s since 1904-01-01), "I_Index"=array[12500 elements], "Q_Index"=array[12500 elements], "10MHz"=FALSE}, "Time"=[], "Saturat"={"MeasMean0"=0.0, "MeasMean1"=0.0, "MeasMax"=0.0, "1_Max"=0.0, "4_Max"=0.0, "5_Max"=0.0, "6_Max"=0.0, "7_Max"=0.0}}} ("cluster")
        # "This is what we were using when we were logging 1 sample at a time.\n-Luke 12/5/2018"
        # "Cluster defined\n in Data_Send"
        # "Write a single Tone record (72Co, 72X, 84Co, 84X)"
        n20 = Variant To Data(error in=w66, type=T30 {"Count"=0, "CalVal"=[], "CalLoc"=[], "BeacVal"=[], "BeacLoc"=[], "BeacShift"=[], "Enum"=enum."1", "df"=0.0, "PwrSpectr"=[], "ISpectr"=[], "QSpectr"=[], "Time"=[], "SNR"=[], "AboveThresh"=[], "10Hz_PeakVal"=[], "Phase"=[], "DeltaPhase"=[], "Saturat"={"Meas"=[], "Stage1"=[], "Stage4"=[], "Stage5"=[], "Stage6"=[], "Stage7"=[]}, "10MHz"=FALSE} ("72co"), Variant=w65) -> (data=w58:T30, error out=w57:errorcluster)
        n21 = call "ChangeFile.vi"("LogLoopClust"=w64) -> ("LogLoopClust out"=w62:T2)  [unwired: 10 in]
        n22 = Unbundle By Name(w62) -> ("LogData.Tone"=w60:T30[])
        n23 = Build Array (concatenate)(w60, w58) -> (w59:T30[])
        n24 = Bundle By Name(cluster=w62, "LogData.Tone"=w59) -> (w61:T2)
      }
      frame "Log_TC" {
        # "Cluster defined\n in Data_Send"
        # "Write a cluster of all TC values with timestamp"
        n25 = call "ChangeFile.vi"("LogLoopClust"=w73) -> ("LogLoopClust out"=w72:T2)  [unwired: 10 in]
        n26 = Variant To Data(error in=w75, type=T49 {"TCData"={"TimeStamp"=0.0, "TimeString"="", "TC0_LP1_Hi"=0.0, "TC1_LP1_MidHi"=0.0, "TC2_LP1_Mid"=0.0, "TC3_LP1_LoMid"=0.0, "TC4_LP1_Lo"=0.0, "TC5_LP2_Hi"=0.0, "TC6_LP2_MidHi"=0.0, "TC7_LP2_Mid"=0.0, "TC8_LP2_LoMid"=0.0, "TC9_LP2_Lo"=0.0, "TC10_HVAC_Cond_In"=0.0, "TC11_HVAC_Cond_Out"=0.0, "TC12_Gen_Exhaust"=0.0, "TC13_Amb_Inter"=0.0, "TC14_Unused"=0.0, "TC15_Unused"=0.0, "TC16_Unused"=0.0, "TC17_Unused"=0.0, "TC18_Unused"=0.0, "TC19_Unused"=0.0, "TC20_Unused"=0.0, "TC21_Unused"=0.0, "TC22_Unused"=0.0, "TC23_Unused"=0.0, "TC24_Unused"=0.0, "TC25_Unused"=0.0, "TC26_Unused"=0.0, "TC27_Unused"=0.0, "TC28_Unused"=0.0, "TC29_Unused"=0.0, "TC30_Unused"=0.0, "TC31_Unused"=0.0}, "All_TC_ErrorStatus"={"TC 0"={"RX?"=FALSE, "Warn"=FALSE, "Error"=FALSE, "Enabl"=FALSE, "Source"=""}, "TC 1"={"RX?"=FALSE, "Warn"=FALSE, "Error"=FALSE, "Enabl"=FALSE, "Source"=""}, "TC 2"={"RX?"=FALSE, "Warn"=FALSE, "Error"=FALSE, "Enabl"=FALSE, "Source"=""}, "TC 3"={"RX?"=FALSE, "Warn"=FALSE, "Error"=FALSE, "Enabl"=FALSE, "Source"=""}, "TC 4"={"RX?"=FALSE, "Warn"=FALSE, "Error"=FALSE, "Enabl"=FALSE, "Source"=""}, "TC 5"={"RX?"=FALSE, "Warn"=FALSE, "Error"=FALSE, "Enabl"=FALSE, "Source"=""}, "TC 6"={"RX?"=FALSE, "Warn"=FALSE, "Error"=FALSE, "Enabl"=FALSE, "Source"=""}, "TC 7"={"RX?"=FALSE, "Warn"=FALSE, "Error"=FALSE, "Enabl"=FALSE, "Source"=""}, "TC 8"={"RX?"=FALSE, "Warn"=FALSE, "Error"=FALSE, "Enabl"=FALSE, "Source"=""}, "TC 9"={"RX?"=FALSE, "Warn"=FALSE, "Error"=FALSE, "Enabl"=FALSE, "Source"=""}, "TC 10"={"RX?"=FALSE, "Warn"=FALSE, "Error"=FALSE, "Enabl"=FALSE, "Source"=""}, "TC 11"={"RX?"=FALSE, "Warn"=FALSE, "Error"=FALSE, "Enabl"=FALSE, "Source"=""}, "TC 12"={"RX?"=FALSE, "Warn"=FALSE, "Error"=FALSE, "Enabl"=FALSE, "Source"=""}, "TC 13"={"RX?"=FALSE, "Warn"=FALSE, "Error"=FALSE, "Enabl"=FALSE, "Source"=""}, "TC 14"={"RX?"=FALSE, "Warn"=FALSE, "Error"=FALSE, "Enabl"=FALSE, "Source"=""}, "TC 15"={"RX?"=FALSE, "Warn"=FALSE, "Error"=FALSE, "Enabl"=FALSE, "Source"=""}, "TC 16"={"RX?"=FALSE, "Warn"=FALSE, "Error"=FALSE, "Enabl"=FALSE, "Source"=""}, "TC 17"={"RX?"=FALSE, "Warn"=FALSE, "Error"=FALSE, "Enabl"=FALSE, "Source"=""}, "TC 18"={"RX?"=FALSE, "Warn"=FALSE, "Error"=FALSE, "Enabl"=FALSE, "Source"=""}, "TC 19"={"RX?"=FALSE, "Warn"=FALSE, "Error"=FALSE, "Enabl"=FALSE, "Source"=""}, "TC 20"={"RX?"=FALSE, "Warn"=FALSE, "Error"=FALSE, "Enabl"=FALSE, "Source"=""}}}, Variant=w74) -> (data=w67:T49, error out=w69:errorcluster)
        n27 = Unbundle By Name(w67) -> ("TCData"=w70:T32)
        n28 = Bundle By Name(cluster=w72, "LogData.TCData"=w70) -> (w71:T2)
      }
      frame "Log_AI" {
        n29 = call "ChangeFile.vi"("LogLoopClust"=w82) -> ("LogLoopClust out"=w81:T2)  [unwired: 10 in]
        n30 = Variant To Data(error in=w84, type=T51 {"AI"={"TimeString"="", "Time Stamp"=0.0, "AI0_Unused"=0.0, "AI1_-5V"=0.0, "AI2_+5V"=0.0, "AI3_+6V"=0.0, "AI4_+12V"=0.0, "AI5_+15V"=0.0, "AI6_+28V"=0.0, "AI7_Unused"=0.0, "Ai16_72GHz_CalPower"=0.0, "Ai17_84GHz_CalPower"=0.0, "Ai18_InclinAz"=0.0, "Ai19_InclinEl"=0.0, "Ai20_BlowerPwr"=0.0, "Ai21_Unused"=0.0, "Ai22_Unused"=0.0, "Ai23_Unused"=0.0, "InclinA_StdDev"=0.0, "InclinB_StdDev"=0.0, "InclinAz_Unfilt"=0.0, "InclinEl_Unfilt"=0.0}, "AllErrorStatus"={"AI 0"={"RX?"=FALSE, "Warn"=FALSE, "Error"=FALSE, "Enabl"=FALSE, "Source"=""}, "AI 1"={"RX?"=FALSE, "Warn"=FALSE, "Error"=FALSE, "Enabl"=FALSE, "Source"=""}, "AI 2"={"RX?"=FALSE, "Warn"=FALSE, "Error"=FALSE, "Enabl"=FALSE, "Source"=""}, "AI 3"={"RX?"=FALSE, "Warn"=FALSE, "Error"=FALSE, "Enabl"=FALSE, "Source"=""}, "AI 4"={"RX?"=FALSE, "Warn"=FALSE, "Error"=FALSE, "Enabl"=FALSE, "Source"=""}, "AI 5"={"RX?"=FALSE, "Warn"=FALSE, "Error"=FALSE, "Enabl"=FALSE, "Source"=""}, "AI 6"={"RX?"=FALSE, "Warn"=FALSE, "Error"=FALSE, "Enabl"=FALSE, "Source"=""}, "AI 7"={"RX?"=FALSE, "Warn"=FALSE, "Error"=FALSE, "Enabl"=FALSE, "Source"=""}, "AI 16"={"RX?"=FALSE, "Warn"=FALSE, "Error"=FALSE, "Enabl"=FALSE, "Source"=""}, "AI 17"={"RX?"=FALSE, "Warn"=FALSE, "Error"=FALSE, "Enabl"=FALSE, "Source"=""}, "AI 18"={"RX?"=FALSE, "Warn"=FALSE, "Error"=FALSE, "Enabl"=FALSE, "Source"=""}, "AI 19"={"RX?"=FALSE, "Warn"=FALSE, "Error"=FALSE, "Enabl"=FALSE, "Source"=""}, "AI 20"={"RX?"=FALSE, "Warn"=FALSE, "Error"=FALSE, "Enabl"=FALSE, "Source"=""}, "AI 21"={"RX?"=FALSE, "Warn"=FALSE, "Error"=FALSE, "Enabl"=FALSE, "Source"=""}, "AI 22"={"RX?"=FALSE, "Warn"=FALSE, "Error"=FALSE, "Enabl"=FALSE, "Source"=""}, "AI 23"={"RX?"=FALSE, "Warn"=FALSE, "Error"=FALSE, "Enabl"=FALSE, "Source"=""}}} ("All_AI"), Variant=w83) -> (data=w77:T51, error out=w78:errorcluster)
        n31 = Unbundle By Name(w77) -> ("AI"=w79:T33)
        n32 = Bundle By Name(cluster=w81, "LogData.AI"=w79) -> (w80:T2)
      }
      frame "Log_DO" {
        # "ch 0: noise\nch 1: 72 GHz Cal\nch 2: 84 GHz Cal"
        n33 = Variant To Data(error in=w90, type=bool[] [] ("appended array"), Variant=w88) -> (data=w85:bool[], error out=w91:errorcluster)
        n34 = Bundle By Name(cluster=w86, "DO"=w85) -> (w87:T2)
      }
      frame "Log_NoiseTrace" {
        # "Cluster defined in Noise_Send"
        n35 = call "ChangeFile.vi"("LogLoopClust"=w98) -> ("LogLoopClust out"=w94:T2)  [unwired: 10 in]
        n36 = Variant To Data(error in=w101, type=cluster{"Target":T13, "NoiseTrace":dbl[]} {"Target"=enum."1", "NoiseTrace"=[]} ("cluster"), Variant=w100) -> (data=w92:cluster{"Target":T13, "NoiseTrace":dbl[]}, error out=w99:errorcluster)
        n37 = Unbundle By Name(w94) -> ("LogData.NoiseTrace"=w93:cluster{"Target":T13, "NoiseTrace":dbl[]}[])
        n38 = Build Array (concatenate)(w93, w92) -> (w95:cluster{"Target":T13, "NoiseTrace":dbl[]}[])
        n39 = Bundle By Name(cluster=w94, "LogData.NoiseTrace"=w95) -> (w96:T2)
      }
      frame "Log_NoiseSum" {
        # "Cluster defined in Noise_Send"
        n40 = call "ChangeFile.vi"("LogLoopClust"=w109) -> ("LogLoopClust out"=w104:T2)  [unwired: 10 in]
        n41 = Variant To Data(error in=w111, type=cluster{"Target":T13, "HDF5_NoiseInfo":T34} {"Target"=enum."1", "HDF5_NoiseInfo"={"Timestring"="Timestamp string goes here", "Timestamp"=0.0, "df"=7629.39453125, "Sum"=0.0}} ("cluster"), Variant=w110) -> (data=w102:cluster{"Target":T13, "HDF5_NoiseInfo":T34}, error out=w107:errorcluster)
        n42 = Unbundle By Name(w104) -> ("LogData.NoiseInfo"=w103:cluster{"Target":T13, "HDF5_NoiseInfo":T34}[])
        n43 = Build Array (concatenate)(w103, w102) -> (w105:cluster{"Target":T13, "HDF5_NoiseInfo":T34}[])
        n44 = Bundle By Name(cluster=w104, "LogData.NoiseInfo"=w105) -> (w106:T2)
      }
      frame "Log_Disdrom" {
        n45 = call "ChangeFile.vi"("LogLoopClust"=w119) -> ("LogLoopClust out"=w114:T2)  [unwired: 10 in]
        n46 = Variant To Data(error in=w121, type=T35 {"Spectrum Data"=[], "DisdromSummary"={"current time"=0.0, "Timestamp"=0.0, "Total Rain Rate"=0.0, "Liquid Rain Rate"=0.0, "Solid Rain Rate"=0.0, "Total Rainfall"=0.0, "Visibility"=0.0, "Radar Reflectivity"=0.0, "Max Diameter Hail"=0.0, "Measured Particles"=0, "Particle Min Speed"=0, "Particle Max Speed"=0, "Particle Min Diam"=0, "NonHydr Particles"=0, "NonHydr Volume"=0.0, "Unkn Particles"=0, "Unkn Volume"=0.0, "HydroType"=0}, "Status"={"Laser"=TRUE, "Signal"=TRUE, "LaserTemp_Analog"=TRUE, "LaserTemp_Digital"=TRUE, "LaserCurrent_Analog"=TRUE, "LaserCurrent_Digital"=TRUE, "SensorSupply"=TRUE, "HeatLaserHead"=TRUE, "HeatReceiverHead"=TRUE, "TempSensor"=TRUE, "HeatSupply"=TRUE, "HeatHousing"=TRUE, "HeatHeads"=TRUE, "HeatCarriers"=TRUE, "OutputLaserPower"=TRUE, "Checksum"=TRUE, "StatusInt"=0}}, Variant=w120) -> (data=w112:T35, error out=w117:errorcluster)
        n47 = Unbundle By Name(w114) -> ("LogData.Disdrom"=w116:T35[])
        n48 = Build Array (concatenate)(w116, w112) -> (w115:T35[])
        n49 = Bundle By Name(cluster=w114, "LogData.Disdrom"=w115) -> (w113:T2)
      }
      frame "Log_Weather" {
        # "Cluster defined\n in Data_Send"
        n50 = Variant To Data(error in=w131, type=T38 {"TimeString"="", "Timestamp"=0.0, "Wind Speed"=0.0, "Wind Gusts"=0.0, "Wind Dir"=0.0, "Wind Dir STD"=0.0, "Temperature"=0.0, "Humidity"=0.0, "Pressure"=0.0, "Rain Rate"=0, "Rain Fall"=0.0, "Status"={"Temp_OutOfBounds"=FALSE, "Temp_IncrSTD"=FALSE, "Temp_Oth"=FALSE, "BarPress_OutOfBounds"=FALSE, "BarPress_IncrSTD"=FALSE, "BarPress_Change"=FALSE, "BarPress_Other"=FALSE, "Humid_OutOfBounds"=FALSE, "Humid_IncrSTD"=FALSE, "Humid_Other"=FALSE, "Wind__Spd_OutOfBounds"=FALSE, "Wind_Dir_OutOfBounds"=FALSE, "RainBuck_OutOfBounds"=FALSE, "RainBuck_Disdrom"=FALSE, "Disdrom_RainBuck"=FALSE, "Placeholder"=FALSE}}, Variant=w130) -> (data=w123:T38, error out=w127:errorcluster)
        n51 = call "ChangeFile.vi"("LogLoopClust"=w129) -> ("LogLoopClust out"=w125:T2)  [unwired: 10 in]
        n52 = Unbundle By Name(w125) -> ("LogData.Weath"=w124:T38[])
        n53 = Build Array (concatenate)(w124, w123) -> (w122:T38[])
        n54 = Bundle By Name(cluster=w125, "LogData.Weath"=w122) -> (w126:T2)
      }
      frame "Log_TE" {
        n55 = call "ChangeFile.vi"("LogLoopClust"=w137) -> ("LogLoopClust out"=w134:T2)  [unwired: 10 in]
        n56 = Variant To Data(error in=w139, type=T40 {"TimeString"="", "TimeStamp"=0.0, "Temp"=0.0, "Output"=0.0, "Temp 2"=0.0, "Output 2"=0.0, "Temp 3"=0.0, "Output 3"=0.0}, Variant=w138) -> (data=w132:T40, error out=w136:errorcluster)
        n57 = Bundle By Name(cluster=w134, "LogData.TE"=w132) -> (w133:T2)
      }
      frame "Log_ADAM" {
        n58 = call "ChangeFile.vi"("LogLoopClust"=w145) -> ("LogLoopClust out"=w142:T2)  [unwired: 10 in]
        n59 = Variant To Data(error in=w147, type=T41 {"Timestamp"=0.0, "Time string"="", "Fault 1"=FALSE, "Fault 2"=FALSE, "Fault 3"=FALSE, "Fault 4"=FALSE, "Fault 5"=FALSE, "Fault 6"=FALSE, "Value 1"=0.0, "Value 2"=0.0, "Value 3"=0.0, "Value 4"=0.0, "Value 5"=0.0, "Value 6"=0.0} ("HealthData"), Variant=w146) -> (data=w140:T41, error out=w144:errorcluster)
        n60 = Bundle By Name(cluster=w142, "LogData.ADAM"=w140) -> (w141:T2)
      }
      frame "Log_UPS" {
        n61 = call "ChangeFile.vi"("LogLoopClust"=w151) -> ("LogLoopClust out"=w150:T2)  [unwired: 10 in]
        n62 = Variant To Data(error in=w153, type=T53 {"Prsnt?"=FALSE, "V"=0.0, "A"=0.0, "Hz"=0.0, "W"=0.0, "%"=0.0, "TimeStamp"=0.0, "TimeString"=""} ("UPS"), Variant=w152) -> (error out=w148:errorcluster)  [unwired: 1 out]
        n63 = Unbundle By Name(w150) -> ()  [unwired: 1 out]
      }
      frame "Log_ChkTime" {
        # "Must check alarm before write case erases data"
        # "Do not write to file if path isn't defined."
        # "Control data log rate. (Write to file once each minute.)"
        # "If still the same minute\ncheck time again."
        # "If not, write data to file"
        # "Is it the same minute as last time?"
        # "What minute is it?"
        n64 = Get Date/Time In Seconds() -> (seconds since 1Jan1904=w155:timestamp)
        n65 = Unbundle By Name(w162) -> ("PathNow1"=w160:path)
        n66 = Format Date/Time String(time format string (%c)="%S", seconds (now)=w155) -> (date/time string=→"date/time string":string)  [unwired: 1 in]
        n67 = Format Date/Time String(time format string (%c)="%M", seconds (now)=w155) -> (date/time string=w169:string)  [unwired: 1 in]
        n68 = Fract/Exp String To Number(string=w169) -> (number=w163:dbl)  [unwired: 3 in, 1 out]
        n69 = Empty String/Path?(string/path=w160) -> (empty?=w159:bool)
        n70 = Not(x=w159) -> (.not. x?=w158:bool)
        n71 = feedback-in #1(w163) -> ()
        n72 = feedback #1(w163) -> (w168:dbl)
        n73 = Not Equal?(x=w163, y=w168) -> (x != y?=w161:bool)
        n74 = And(x=w158, y=w161) -> (x .and. y?=w157:bool)
        n75 = Select(t=cluster{"Enum":T1, "Data":variant}[] [{"Enum"=enum."Log_Alarm", "Data"=variant}, {"Enum"=enum."Log_SSH", "Data"=variant}, {"Enum"=enum."Log_Write", "Data"=variant}, {"Enum"=enum."Log_ChkTime", "Data"=variant}] ("element"), s=w157, f=cluster{"Enum":T1, "Data":variant}[] [{"Enum"=enum."Log_ChkTime", "Data"=variant}] ("element")) -> (s? t:f=w164:cluster{"Enum":T1, "Data":variant}[])
        n76 = for {
          tunnel: w172 -> [w176]
          tunnel: w164 -> [w174] mode=indexing
          shift-right: [w177] -> w173
          shift-left: w171 -> [w175]
          n77 = Enqueue Element(queue=w176, element=w174, error in (no error)=w175) -> (error out=w177:errorcluster)  [unwired: 1 in, 2 out]
        }
        n78 = Wait (ms)(milliseconds to wait=u32 50) -> ()  [unwired: 1 out]
      }
      frame "Log_Alarm" {
        w196 = cluster{"Enum":T59, "Data":variant} {"Enum"=enum."FP_Alarm", "Data"=variant}
        # "Don't send alarm\nuntil 15 minutes,\nto allow all signals\nto settle."
        # "Send to FP for display\nSend to DO for actual HW signal"
        n79 = call "Alarm_CompareToThresholds.vi"("HDF5_file_refs"=w184) -> ("AllAlarms"=w183:T45[], "Alarm Status"=w178:T46, "WeatherStatus"=w181:bool[], "Elapsed_SNR_Timer"=w180:dbl, "SaturationStatus"=w179:T47)  [unwired: 6 in]
        n80 = call "Elapsed Time"("Time Target (s)"=900.0, "error in (no error)"=w190) -> ("Time has Elapsed"=w188:bool, "error out"=w189:errorcluster)  [unwired: 10 in, 6 out]
        n81 = Bundle By Name(cluster=w184, "SaturationStatus"=w179, "WeatherStatus"=w181, "Alarm Status"=w178, "AllAlarms"=w183) -> (w185:T2)
        n82 = call "Sort_FP_Alarm.vi"("Alarm Status"=w178, "Elapsed_SNR_Timer"=w180, "AllAlarms"=w183, "HDF5_file_refs"=w184) -> ("AlarmDisplay"=w186:T60)  [unwired: 7 in]
        n83 = case shown="True" w188 {
          tunnel: [errorcluster {"status"=FALSE, "code"=0, "source"=""} ("error out") w207] -> w191
          tunnel: w178 -> [_ w206]
          frame False {
          }
          frame True {
            w211 = cluster{"Enum":T62, "Data":variant} {"Enum"=enum."Digi_Write", "Data"=variant}
            n84 = Obtain Queue(max queue size (-1, unlimited)=100, name (unnamed)="Digi", element data type=w211) -> (queue out=w214:refnum<queue>, error out=w210:errorcluster)  [unwired: 2 in, 1 out]
            n85 = To Variant(anything=w206) -> (Variant=w213:variant)
            n86 = Bundle By Name(cluster=w211, "Data"=w213) -> (w212:cluster{"Enum":T62, "Data":variant})
            n87 = Enqueue Element(queue=w214, element=w212, timeout in ms (-1)=10, error in (no error)=w210) -> (queue out=w208:refnum<queue>, error out=w209:errorcluster)  [unwired: 1 out]
            n88 = Release Queue(queue=w208, error in (no error)=w209) -> (error out=w207:errorcluster)  [unwired: 1 in, 2 out]
          }
        }
        n89 = Obtain Queue(name (unnamed)="FP", element data type=w196) -> (queue out=w198:refnum<queue>, error out=w199:errorcluster)  [unwired: 3 in, 1 out]
        n90 = To Variant(anything=w186) -> (Variant=w197:variant)
        n91 = Bundle By Name(cluster=w196, "Data"=w197) -> (w200:cluster{"Enum":T59, "Data":variant})
        n92 = Enqueue Element(queue=w198, element=w200, timeout in ms (-1)=10, error in (no error)=w199) -> (queue out=w202:refnum<queue>, error out=w201:errorcluster)  [unwired: 1 out]
        n93 = Release Queue(queue=w202, error in (no error)=w201) -> (error out=w192:errorcluster)  [unwired: 1 in, 2 out]
        n94 = Merge Errors(w192, w191, w189) -> (w193:errorcluster)
        n95 = call "PushToErrorHandler.vi"("ErrorIn"=w193, "ErrorLocation"="Log") -> ("ErrorOut"=w194:errorcluster)  [unwired: 5 in]
      }
      frame "Log_SSH" {
        # "TCP string is written in TCP Loop"
        n96 = flat-sequence {
          tunnel: [w232] -> w222
          tunnel: [w231] -> w224
          frame #0 {
            w232 = "192.168.2.1"  # WSCEr_IP_Addr
            n97 = Tick Count (ms)() -> (millisecond timer value=w231:u32)
          }
        }
        n98 = call "Watchdog_Functional_Global.vi"("Watchdog"=WatchdogTimer_Enum."CheckAll") -> (2:"Elapsed"=w217:string, 5:"Elapsed"=→"WatchDogElapsed":i32[])  [unwired: 8 in, 1 out]
        n99 = disable-structure shown="Enabled" {
          disable-tunnel: [w236 w241] -> w220
          disable-tunnel: w222 -> [_ w239]
          disable-tunnel: w221 -> [w235 w238]
          disable-tunnel: w217 -> [w233 _]
          frame Enabled {
            n100 = call "Build_TCP_String.vi"("WatchdogString"=w233, "LogLoopClust"=w235) -> ("TCP string"=w234:string)  [unwired: 9 in]
            n101 = shared-variable ".\\Connex_Variables.lvlib\\TCP_String"(w234) -> (error out=w236:errorcluster)  [unwired: 1 in]
          }
          frame Disabled {
            w244 = TRUE  # run minimized? (F)
            n102 = call "Build_SSH_String.vi"("WSCEr_IP_Addr"=w239, "LogLoopClust"=w238) -> ("SSH_String"=w237:string)  [unwired: 8 in, 1 out]
            n103 = call <vilib>:"System Exec.vi"("run minimized? (F)"=w244, "wait until completion? (T)"=FALSE, "command line"=w237) -> ("error out"=w242:errorcluster)  [unwired: 5 in, 3 out]
            n104 = Unbundle By Name(w242) -> ()  [unwired: 1 out]
            n105 = call "PushToErrorHandler.vi"("ErrorIn"=w242, "ErrorLocation"="SSH") -> ("ErrorOut"=w241:errorcluster)  [unwired: 5 in]
          }
        }
        n106 = flat-sequence {
          tunnel: [w230] -> w225
          tunnel: w220 -> [w230]
          tunnel: w224 -> [w228]
          tunnel: [w227] -> w223
          frame #0 {
            n107 = Tick Count (ms)() -> (millisecond timer value=w229:u32)
            n108 = Subtract(x=w229, y=w228) -> (x-y=w227:u32)
          }
        }
        "Elapsed" <- w223
      }
      frame "Log_Write" {
        # "Reset\nWatchdog"
        n109 = call "ChangeFile.vi"("LogLoopClust"=w247) -> ("LogLoopClust out"=w246:T2)  [unwired: 10 in]
        n110 = call "Log_WriteToFile.vi"("error in"=w251, "LogClust"=w246) -> ("ErrorOut"=w249:errorcluster, "HDF5_file_refs"=w245:T2)  [unwired: 8 in]
        n111 = call "Watchdog_Functional_Global.vi"("Watchdog"=WatchdogTimer_Enum."Log", "error in"=w249) -> ("error out"=w248:errorcluster)  [unwired: 7 in, 2 out]
      }
      frame "Log_Exit" {
        w252 = 60004 ("specific error code to clear (0: all)")
        # "Error 6004 is expected if the file hasn't been\ncreated yet."
        # "Close HDF5 files"
        n112 = Release Queue(queue=w265, error in (no error)=w264) -> (error out=w260:errorcluster)  [unwired: 1 in, 2 out]
        n113 = Unbundle By Name(w261) -> ("HDFRefs1.File"=w257:T15, "HDFRefs2.File"=w262:T15)
        n114 = call "PushToErrorHandler.vi"("ErrorIn"=w260, "ErrorLocation"="LogExit") -> ("ErrorOut"=w259:errorcluster)  [unwired: 5 in]
        n115 = call <vilib>:"H5Fclose.vi"("error in (no error)"=w259, "ref"=w262) -> ("error out"=w256:errorcluster)  [unwired: 9 in]
        n116 = call <vilib>:"Clear Errors.vi"("error in (no error)"=w256, "specific error code to clear (0: all)"=w252) -> ("error out"=w255:errorcluster)  [unwired: 4 in, 1 out]
        n117 = call <vilib>:"H5Fclose.vi"("error in (no error)"=w255, "ref"=w257) -> ("error out"=w254:errorcluster)  [unwired: 9 in]
        n118 = call <vilib>:"Clear Errors.vi"("error in (no error)"=w254, "specific error code to clear (0: all)"=w252) -> ("error out"=w253:errorcluster)  [unwired: 4 in, 1 out]
      }
      frame Default {
        "Enum" <- w267
      }
    }
    n119 = call "FileFailed.vi"("error in (no error)"=w10, "HDF5_file_refs in"=w6) -> ("error out"=w14:errorcluster, "HDF5_file_refs out"=w13:T2)  [unwired: 8 in]
    "LogCount" <- w9
  }
  "error out" <- w3
